vi "HMI_Prototype.vi"() -> ()   [LabVIEW 2015]
uses:
  System.Windows.Forms
  machineState.ctl
  controls.ctl
  <vilib>/DAQmx/write.llb/DAQmx Write (Digital Bool 1Line 1Point).vi
  <vilib>/DAQmx/read.llb/DAQmx Read (Analog DBL 1Chan 1Samp).vi
  <vilib>/DAQmx/miscellaneous.llb/DAQmx Fill In Error Info.vi
panel:
  out "lab":dbl
  out "solution":dbl
  out "Issue Resolved:":bool
  out "Budget:":dbl=800.0 format="$%#_g.00"
  out "Time Remaining:":timestamp=timestamp(1800 s since 1904-01-01) format="%<%M:%S>T"
  in  "Terminal:":T1(ring)
  in  "Component:":T2(ring)
  in  "Tighten Terminal":bool
  in  "Replace Component":bool
  in  "Segment:":T3(ring)
  in  "Aquire Voltage":bool
  out "Voltage:":dbl
  out "Lab:":string
  in  "Close Lab":bool
  in  "Reset Lab":bool
  out "B+ Solenoid":bool
  out "A- Solenoid":bool
  out "A+ Solenoid":bool
  out "Manual":bool
  out "Auto":bool=TRUE
  out "Stop Button":bool
  out "Start Button":bool
  in  "Tab Control":T4(tab)
  in  "WebBrowser":refnum<k7>(container)
  in  "Schematic1":refnum<k24>(container)
  in  "Schematic2":refnum<k24>(container)
  in  "Schematic3":refnum<k24>(container)
  in  "Schematic4":refnum<k24>(container)
  in  "B+":bool
  in  "A-":bool
  in  "A+":bool
  in  "START":bool
  in  "AUTO/MAN":bool
  in  "STOP":bool
  # "A+"
  # "A-"
  # "B+"
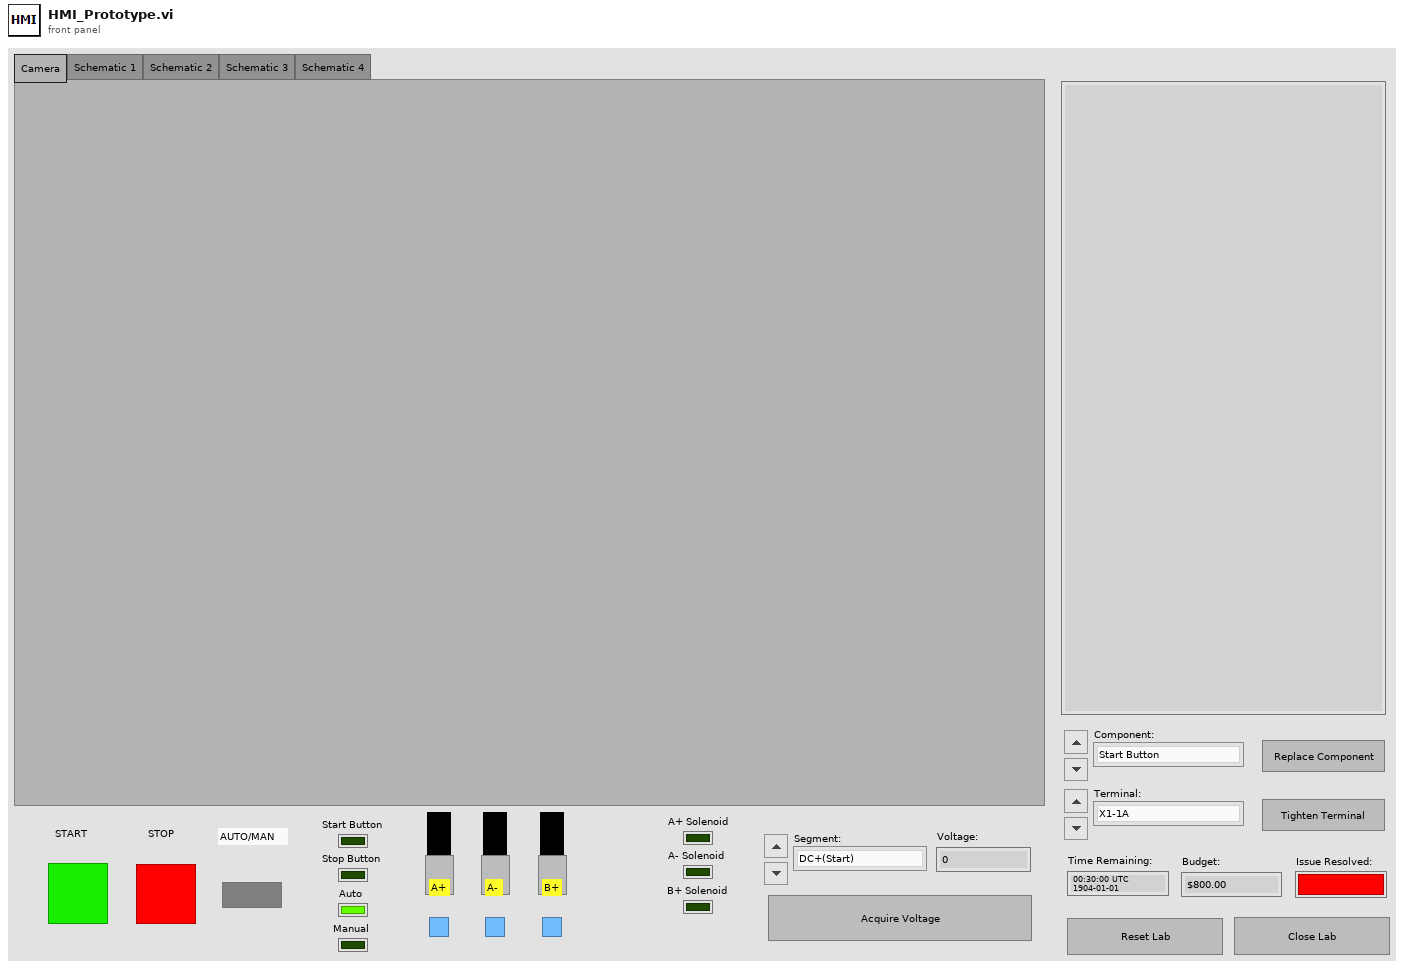
[diagram p1: front panel]
types:
  T1 = enum16{"X1-1A", "X1-2A", "X1-3A", "X1-4A", "X1-5A", "X1-6A", "X1-7A", "X1-8A", "X1-9A", "X1-10A", "X1-11A", "X1-12A", "X1-1B", "X1-2B", "X1-3B", "X1-4B", "X1-5B", "X1-6B", "X1-7B", "X1-8B", "X1-9B", "X1-10B", "X1-11B", "X1-12B", "X1-1C", "X1-2C", "X1-3C", "X1-4C", "X1-5C", "X1-6C", "X1-7C", "X1-8C", "X1-9C", "X1-10C", "X1-11C", "X1-12C", "X1-1D", "X1-2D", "X1-3D", "X1-4D", "X1-5D", "X1-6D", "X1-7D", "X1-8D", "X1-9D", "X1-10D", "X1-11D", "X1-12D", "PLC-VDC(O/0)", "PLC-O/0", "PLC-VDC(O/1)", "PLC-O/1", "PLC-VDC(O/2)", "PLC-O/2", "PLC-VDC(O/3)", "PLC-O/3", "PLC-DC_COM1", "PLC-I/0", "PLC-I/1", "PLC-I/2", "PLC-I/3", "PLC-DC_COM2", "PLC-I/4", "PLC-I/5", "PLC-I/6", "PLC-I/7", "Start Button Terminals", "Stop Button Terminals", "Auto/Man Terminals", "DM1(a0) Terminals", "DM2(a1) Terminals", "DM3(b0) Terminals", "DM4(b1) Terminals", "DM5(v) Terminals", "EL1(A+) Terminals", "EL2(A-) Terminals", "EL3(B+) Terminals", "EL4(V+) Terminals"}
  T2 = enum16{"Start Button", "Stop Button", "Auto/Man Switch", "DM1(a0)", "DM2(a1)", "DM3(b0)", "DM4(b1)", "DM5(v)", "EL1(A+)", "EL2(A-)", "EL3(B+)", "EL4(V+)", "PLC"}
  T3 = enum16{"DC+(Start)", "PB(Start)", "I/0(Start)", "DC+(Stop)", "PB(Stop)", "I/1(Stop)", "DC+(Auto/Man)", "I/2(Auto/Man)", "DC+(a0)", "I/3(a0)", "DC+(a1)", "I/4(a1)", "DC+(b0)", "I/5(b0)", "DC+(b1)", "I/6(b1)", "DC+(v)", "I/7(v)", "DC+(O/0)(VAC/VDC)", "O/0(EL1A+)", "EL1A+(A1)", "EL1A+(A2)", "DC+(O/1)(VAC/VDC)", "O/1(EL2A-)", "EL2A-(A1)", "EL2A-(A2)", "O/2(EL3B+)(A1)", "EL3B+(A2)", "O/3(EL4V+)(A1)", "EL4V+(A2)", "DC-(DC_COM)", "DC-(0V)"}
  T4 = enum32{"Camera", "Schematic 1", "Schematic 2", "Schematic 3", "Schematic 4"}
  T5 = typedef "controls.ctl" = enum16{"Initialize", "Start Button", "Stop Button", "AutoMan Switch", "A Plus Button", "A Minus Button", "B Plus Button", "V Plus Button", "Change View", "Acquire Voltage", "Replace Component", "Tighten Terminal", "Reset Lab", "Close Lab"}
  T6 = typedef "machineState.ctl" = enum16{"idle", "running"}
  T7 = enum16{"open", "replace", "create", "open or create", "replace or create", "replace or create with confirmation"}
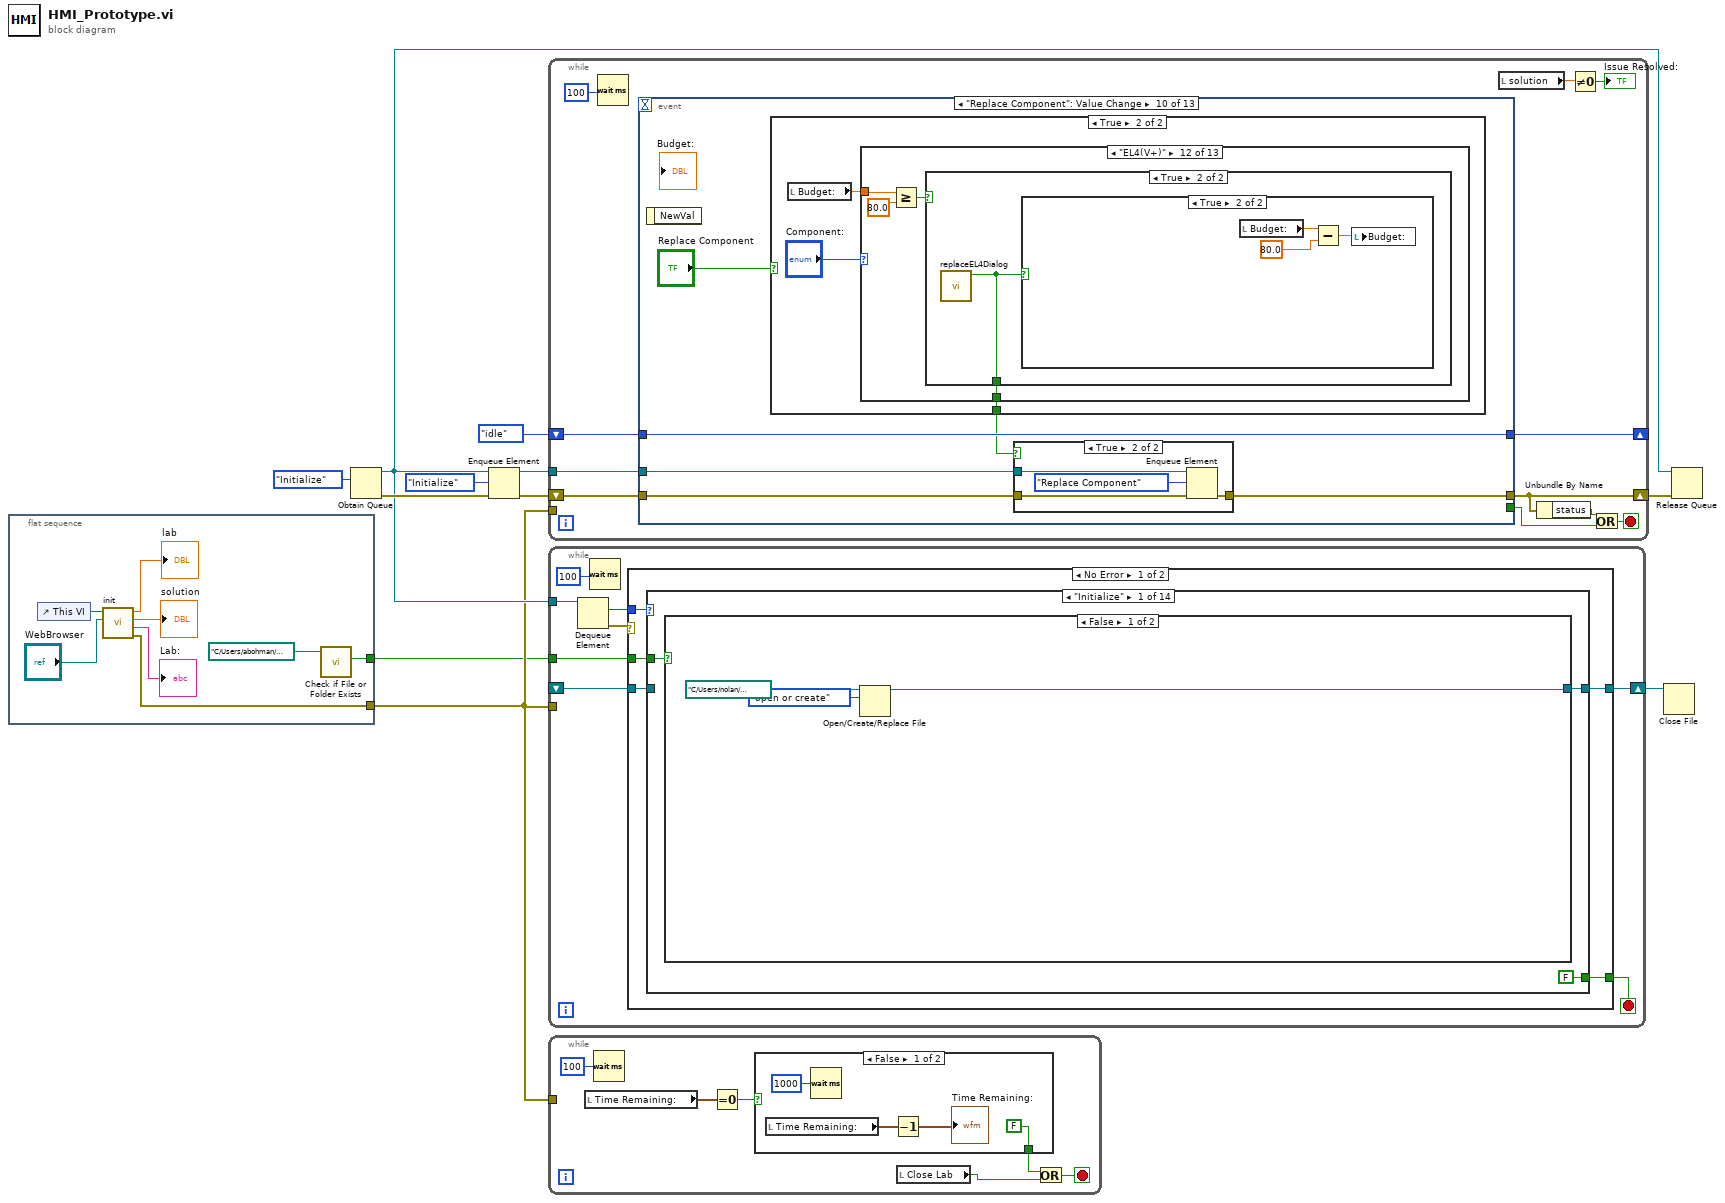
[diagram p0: block diagram]
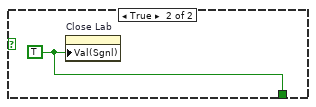
[diagram p2: hidden frame]
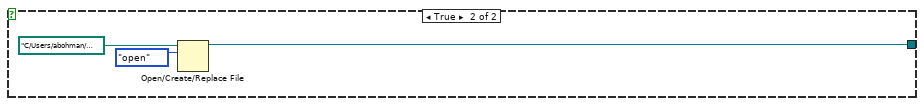
[diagram p3: hidden frame]
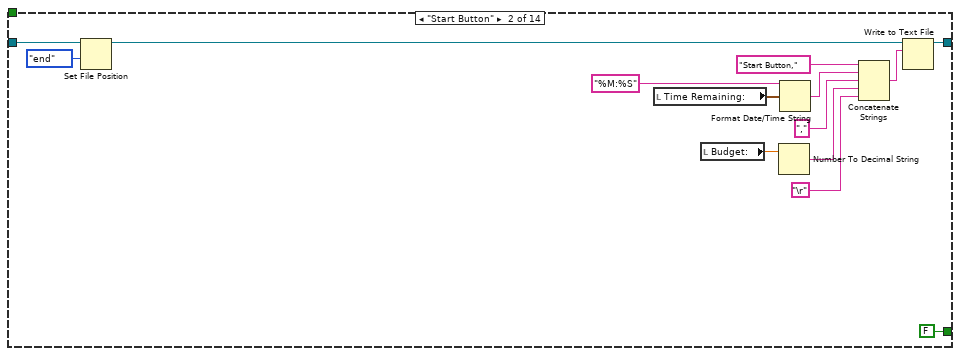
[diagram p4: hidden frame]
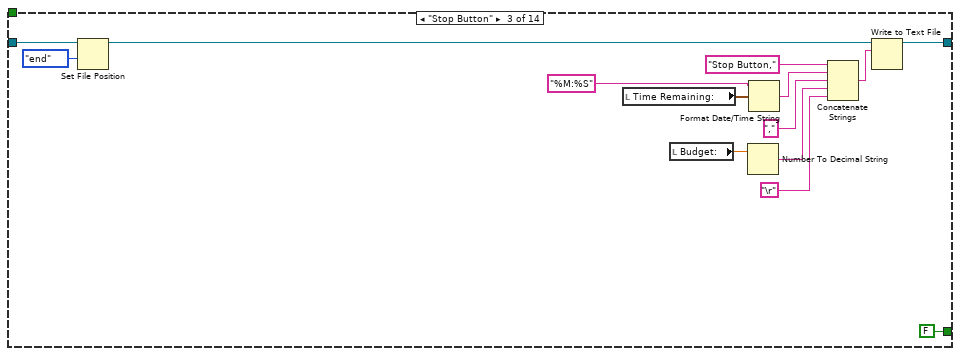
[diagram p5: hidden frame]
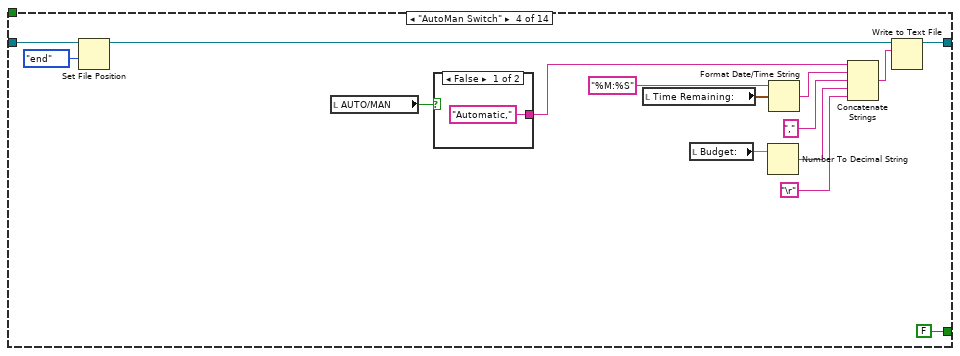
[diagram p6: hidden frame]
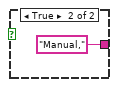
[diagram p7: hidden frame]
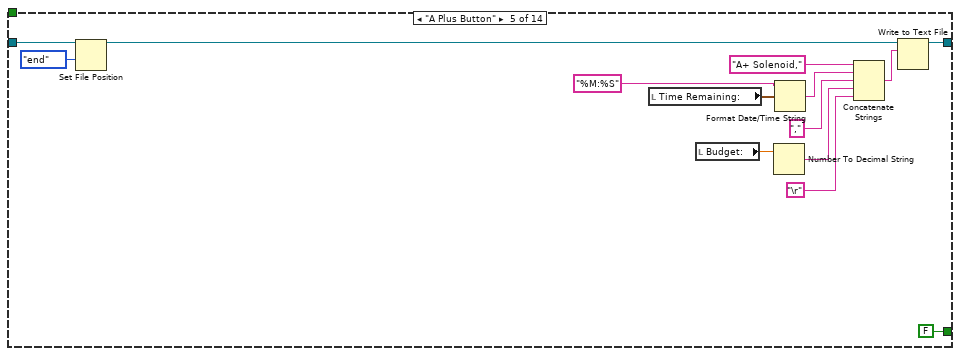
[diagram p8: hidden frame]
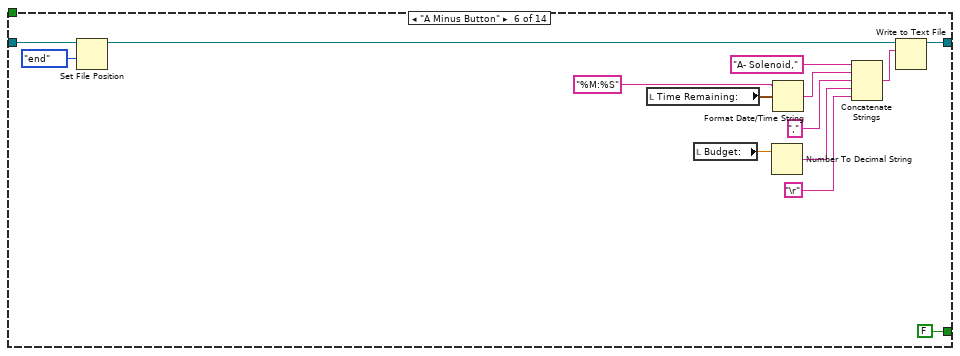
[diagram p9: hidden frame]
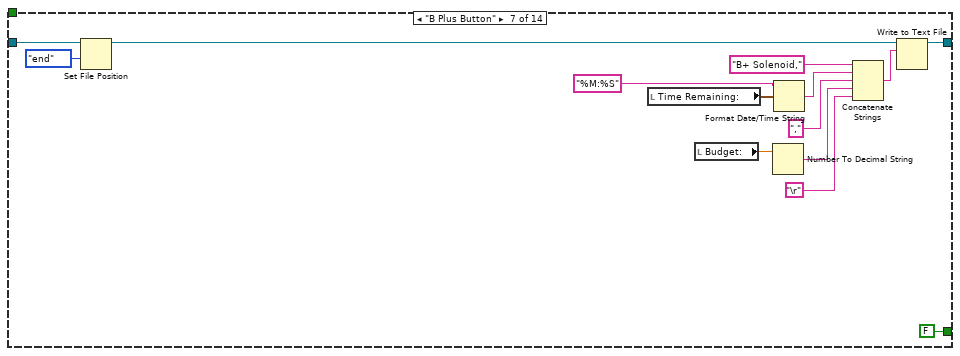
[diagram p10: hidden frame]
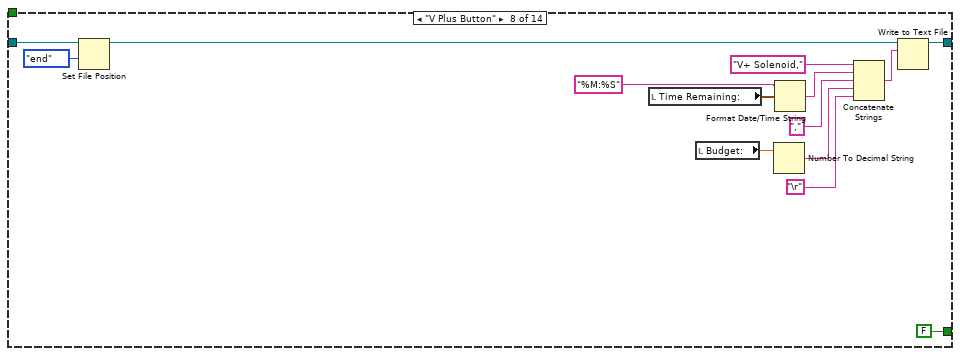
[diagram p11: hidden frame]
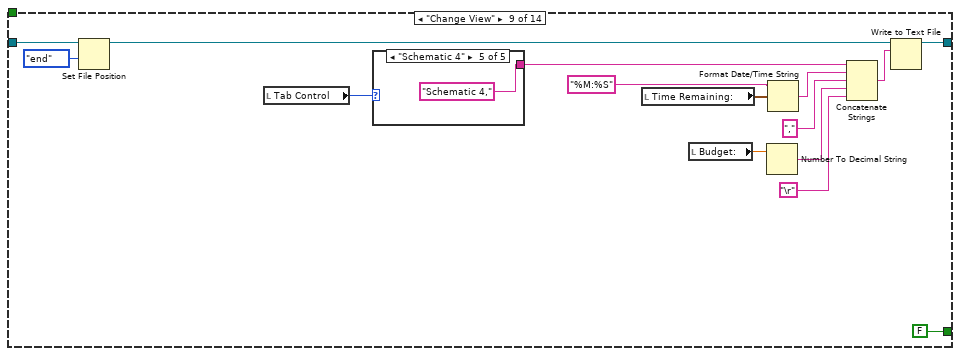
[diagram p12: hidden frame]
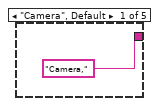
[diagram p13: hidden frame]
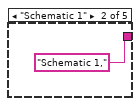
[diagram p14: hidden frame]
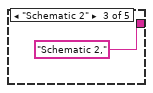
[diagram p15: hidden frame]
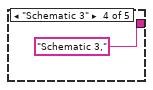
[diagram p16: hidden frame]
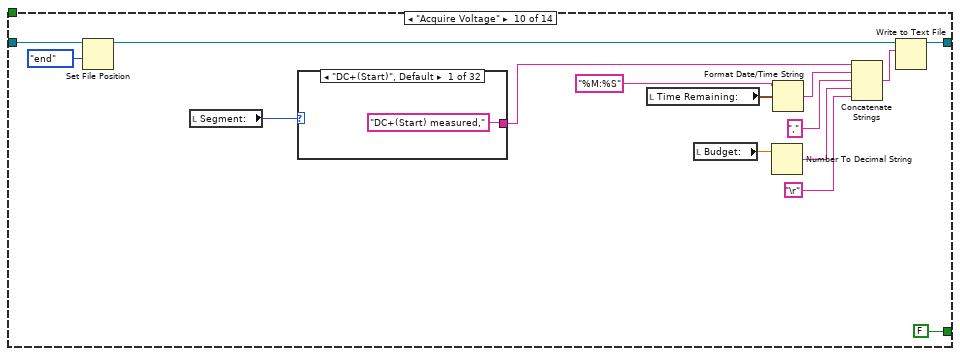
[diagram p17: hidden frame]
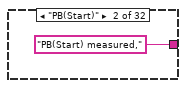
[diagram p18: hidden frame]
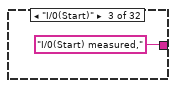
[diagram p19: hidden frame]
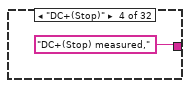
[diagram p20: hidden frame]
diagram:
  n1 = flat-sequence {
    tunnel: [w14] -> w3
    tunnel: [w12] -> w2
    frame #0 {
      n2 = control-ref of="This VI"() -> (w19:refnum<vi>)
      n3 = call "init.vi"("WebBrowser"="WebBrowser", "VI in"=w19) -> ("error out"=w14:errorcluster, "Lab Description:"=→"Lab:":string, "solution"=→"solution":dbl, "lab"=→"lab":dbl)  [unwired: 6 in]
      n4 = call <vilib>:"Check if File or Folder Exists.vi"("path"=path "C:/Users/abohman/Desktop/iMEC-HMI/userLog.txt") -> ("file or folder exists?"=w12:bool)  [unwired: 8 in, 2 out]
    }
  }
  n5 = Obtain Queue(element data type=controls."Initialize") -> (queue out=w4:refnum<queue>, error out=w5:errorcluster)  [unwired: 4 in, 1 out]
  n6 = Enqueue Element(queue=w4, element=controls."Initialize", error in (no error)=w5) -> (queue out=w8:refnum<queue>, error out=w7:errorcluster)  [unwired: 1 in, 1 out]
  n7 = while {
    shift-right: [w25] -> w10
    shift-left: w7 -> [w29]
    tunnel: w8 -> [w28]
    shift-right: [w26] -> _
    shift-left: machineState."idle" -> [w27]
    tunnel: w3 -> [_]
    stop <- w24 stop-if-true
    n8 = Wait (ms)(milliseconds to wait=u32 100 ("millisecond timer value")) -> ()  [unwired: 1 out]
    n9 = event shown="[9] \"Replace Component\": Value Change" {
      selector: _ -> [_ _ _ _ _ _ _ _ _ _ _ _ _]
      dyn-events: _ -> [_ _ _ _ _ _ _ _ _ _ _ _ _]
      timeout: _ -> [_ _ _ _ _ _ _ _ _ _ _ _ _]
      tunnel: w29 -> [w42 w69 w78 w91 w106 w122 w137 w142 w189 w195 w405 w516 w547]
      tunnel: [w41 w68 w79 w90 w105 w121 w136 w141 w189 w194 w404 w515 w545] -> w25
      tunnel: w28 -> [w40 w67 w77 w92 w107 w120 w138 w143 _ w196 w406 w517 w546]
      tunnel: w27 -> [w34 w64 w81 w89 w104 w119 w134 w140 w190 w193 w403 w514 w543]
      tunnel: [w35 w63 w81 w89 w104 w119 w134 w140 w190 w193 w403 w514 w543] -> w26
      tunnel: [_ _ _ _ _ _ _ _ _ _ _ _ w541] -> w22
      event "START": Value Change {
        w37 = refnum<k21> "DO1P0"  # Start Button
        n10 = event-data() -> ("NewVal"=w31:bool)  [unwired: 1 in]
        n11 = local read "AUTO/MAN"() -> (w39:bool)
        n12 = case shown="True" w31 {
          tunnel: w42 -> [w43 w47]
          tunnel: [w43 w46] -> w41
          tunnel: w40 -> [_ w45]
          frame False {
          }
          frame True {
            n13 = Enqueue Element(queue=w45, element=controls."Start Button", error in (no error)=w47) -> (error out=w46:errorcluster)  [unwired: 1 in, 2 out]
          }
        }
        n14 = case shown="False" w39 {
          tunnel: [w50 w60] -> w36
          tunnel: [w51 w59] -> w35
          tunnel: w34 -> [w52 w59]
          tunnel: "START" -> [w48 w60]
          tunnel: [w49 w60] -> w32
          frame False {
            n15 = case shown="\"idle\"" w52 {
              selector: w52 -> [_ w58]
              tunnel: [machineState."running" w58] -> w51
              tunnel: [TRUE ("START") FALSE ("START")] -> w50
              tunnel: [w53 w56] -> w49
              tunnel: w48 -> [w53 w56]
              frame "idle" {
              }
              frame "running" {
              }
            }
          }
          frame True {
          }
        }
        "Start Button" <- w32
        n16 = call-poly <vilib>:"DAQmx Write.vi"("task/channels in"=w37, "data"=w36) -> ("task out"=w38:refnum<k21>)  [unwired: 11 in, 2 out]
        n17 = call <vilib>:"DAQmx Clear Task.vi"("task in"=w38) -> ()  [unwired: 14 in, 1 out]
      }
      event "STOP": Value Change {
        w65 = refnum<k21> "DO1P1"  # Stop Button
        n18 = event-data() -> ("NewVal"=w62:bool)  [unwired: 1 in]
        n19 = case shown="True" w62 {
          tunnel: w69 -> [w70 w74]
          tunnel: [w70 w73] -> w68
          tunnel: w67 -> [_ w72]
          frame False {
          }
          frame True {
            n20 = Enqueue Element(queue=w72, element=controls."Stop Button", error in (no error)=w74) -> (error out=w73:errorcluster)  [unwired: 1 in, 2 out]
          }
        }
        n21 = case shown="\"running\"" w64 {
          selector: w64 -> [w75 _]
          tunnel: [w75 machineState."idle"] -> w63
          frame "idle" {
          }
          frame "running" {
          }
        }
        n22 = call-poly <vilib>:"DAQmx Write.vi"("task/channels in"=w65, "data"="STOP") -> ("task out"=w66:refnum<k21>)  [unwired: 11 in, 2 out]
        n23 = call <vilib>:"DAQmx Clear Task.vi"("task in"=w66) -> ()  [unwired: 14 in, 1 out]
        "Stop Button" <- "STOP"
      }
      event "AUTO/MAN": Value Change {
        n24 = event-data() -> ()  [unwired: 1 in, 1 out]
        n25 = case shown="\"idle\"" w81 {
          frame "idle" {
            w83 = refnum<k21> "DO1P2"  # Auto/Man
            n26 = Equal?(x="AUTO/MAN", y=FALSE) -> (x = y?=→"Auto":bool)
            n27 = call-poly <vilib>:"DAQmx Write.vi"("task/channels in"=w83, "data"="AUTO/MAN") -> ("task out"=w84:refnum<k21>)  [unwired: 11 in, 2 out]
            n28 = call <vilib>:"DAQmx Clear Task.vi"("task in"=w84) -> ()  [unwired: 14 in, 1 out]
            "Manual" <- "AUTO/MAN"
          }
          frame "running" {
            n29 = One Button Dialog(message="The machine is still running.  Please\nstop the machine before switching\nit into 'Manual' mode." ("button name (\"OK\")")) -> ()  [unwired: 1 in, 1 out]
            n30 = invoke on="AUTO/MAN" class="Bool (strict)" method="Reinit To Default"() -> ()  [unwired: 3 in, 3 out]
          }
        }
        n31 = Enqueue Element(queue=w77, element=controls."AutoMan Switch", error in (no error)=w78) -> (error out=w79:errorcluster)  [unwired: 1 in, 2 out]
      }
      event "A+": Value Change {
        n32 = event-data() -> ("NewVal"=w88:bool)  [unwired: 1 in]
        n33 = case shown="True" w88 {
          tunnel: w92 -> [_ w97]
          tunnel: w91 -> [w93 w96]
          tunnel: [w93 w95] -> w90
          frame False {
          }
          frame True {
            n34 = Enqueue Element(queue=w97, element=controls."A Plus Button", error in (no error)=w96) -> (error out=w95:errorcluster)  [unwired: 1 in, 2 out]
          }
        }
        n35 = case shown="\"idle\"" w89 {
          frame "idle" {
            w99 = refnum<k21> "DO1P3"  # A+ Solenoid
            n36 = call-poly <vilib>:"DAQmx Write.vi"("task/channels in"=w99, "data"="A+") -> ("task out"=w100:refnum<k21>)  [unwired: 11 in, 2 out]
            n37 = call <vilib>:"DAQmx Clear Task.vi"("task in"=w100) -> ()  [unwired: 14 in, 1 out]
            "A+ Solenoid" <- "A+"
          }
          frame "running" {
            n38 = local read "A+"() -> (w101:bool)
            n39 = case shown="True" w101 {
              frame False {
              }
              frame True {
                n40 = One Button Dialog(message="The machine is still running. Please\nstop the machine before using\nthe solenoid controls.") -> ()  [unwired: 1 in, 1 out]
              }
            }
          }
        }
      }
      event "A-": Value Change {
        n41 = event-data() -> ("NewVal"=w103:bool)  [unwired: 1 in]
        n42 = case shown="True" w103 {
          tunnel: w107 -> [_ w112]
          tunnel: w106 -> [w108 w111]
          tunnel: [w108 w110] -> w105
          frame False {
          }
          frame True {
            n43 = Enqueue Element(queue=w112, element=controls."A Minus Button", error in (no error)=w111) -> (error out=w110:errorcluster)  [unwired: 1 in, 2 out]
          }
        }
        n44 = case shown="\"idle\"" w104 {
          frame "idle" {
            w114 = refnum<k21> "DO1P4"  # A- Solenoid
            n45 = call-poly <vilib>:"DAQmx Write.vi"("task/channels in"=w114, "data"="A-") -> ("task out"=w115:refnum<k21>)  [unwired: 11 in, 2 out]
            n46 = call <vilib>:"DAQmx Clear Task.vi"("task in"=w115) -> ()  [unwired: 14 in, 1 out]
            "A- Solenoid" <- "A-"
          }
          frame "running" {
            n47 = local read "A-"() -> (w116:bool)
            n48 = case shown="True" w116 {
              frame False {
              }
              frame True {
                n49 = One Button Dialog(message="The machine is still running. Please\nstop the machine before using\nthe solenoid controls.") -> ()  [unwired: 1 in, 1 out]
              }
            }
          }
        }
      }
      event "B+": Value Change {
        n50 = event-data() -> ("NewVal"=w118:bool)  [unwired: 1 in]
        n51 = case shown="True" w118 {
          tunnel: w122 -> [w123 w127]
          tunnel: [w123 w126] -> w121
          tunnel: w120 -> [_ w125]
          frame False {
          }
          frame True {
            n52 = Enqueue Element(queue=w125, element=controls."B Plus Button", error in (no error)=w127) -> (error out=w126:errorcluster)  [unwired: 1 in, 2 out]
          }
        }
        n53 = case shown="\"running\"" w119 {
          frame "idle" {
            w129 = refnum<k21> "DO1P5"  # B+ Solenoid
            n54 = call-poly <vilib>:"DAQmx Write.vi"("task/channels in"=w129, "data"="B+") -> ("task out"=w130:refnum<k21>)  [unwired: 11 in, 2 out]
            n55 = call <vilib>:"DAQmx Clear Task.vi"("task in"=w130) -> ()  [unwired: 14 in, 1 out]
            "B+ Solenoid" <- "B+"
          }
          frame "running" {
            n56 = local read "B+"() -> (w131:bool)
            n57 = case shown="True" w131 {
              frame False {
              }
              frame True {
                n58 = One Button Dialog(message="The machine is still running. Please\nstop the machine before using\nthe solenoid controls.") -> ()  [unwired: 1 in, 1 out]
              }
            }
          }
        }
      }
      event "Tab Control": Value Change {
        n59 = event-data() -> ()  [unwired: 1 in, 1 out]
        n60 = case shown="\"Schematic 1\"" "Tab Control" {
          frame "Camera", Default {
          }
          frame "Schematic 1" {
          }
          frame "Schematic 2" {
          }
          frame "Schematic 3" {
          }
          frame "Schematic 4" {
          }
        }
        n61 = Enqueue Element(queue=w138, element=controls."Change View", error in (no error)=w137) -> (error out=w136:errorcluster)  [unwired: 1 in, 2 out]
      }
      event "Aquire Voltage": Value Change {
        n62 = event-data() -> ("NewVal"=w139:bool)  [unwired: 1 in]
        n63 = while {
          stop <- w149 stop-if-true
          n64 = case shown="True" "Aquire Voltage" {
            tunnel: [TRUE FALSE] -> w149
            frame False {
            }
            frame True {
              n65 = case shown="\"DC-(DC_COM)\"" "Segment:" {
                tunnel: [w157 w158 w159 w160 w161 w162 w163 w164 w165 w166 w167 w168 w169 w170 w171 w172 w173 w174 w175 w176 w177 w178 w179 w180 w181 w182 w183 w184 w185 w186 w187 w188] -> w154
                frame "DC+(Start)" {
                  w157 = refnum<k21> "ACH00"  # DC+(Start)
                }
                frame "PB(Start)" {
                  w158 = refnum<k21> "ACH01"  # PB(Start)
                }
                frame "I/0(Start)" {
                  w159 = refnum<k21> "ACH02"  # I/0(Start)
                }
                frame "DC+(Stop)" {
                  w160 = refnum<k21> "ACH03"  # DC+(Stop)
                }
                frame "PB(Stop)" {
                  w161 = refnum<k21> "ACH04"  # PB(Stop)
                }
                frame "I/1(Stop)" {
                  w162 = refnum<k21> "ACH05"  # I/1(Stop)
                }
                frame "DC+(Auto/Man)" {
                  w163 = refnum<k21> "ACH06"  # DC+(Auto/Man)
                }
                frame "I/2(Auto/Man)" {
                  w164 = refnum<k21> "ACH07"  # I/2(Auto/Man)
                }
                frame "DC+(a0)" {
                  w165 = refnum<k21> "ACH08"  # DC+(A0)
                }
                frame "I/3(a0)" {
                  w166 = refnum<k21> "ACH09"  # I/3(A0)
                }
                frame "DC+(a1)" {
                  w167 = refnum<k21> "ACH10"  # DC+(A1)
                }
                frame "I/4(a1)" {
                  w168 = refnum<k21> "ACH11"  # I/4(A1)
                }
                frame "DC+(b0)" {
                  w169 = refnum<k21> "ACH12"  # DC+(B0)
                }
                frame "I/5(b0)" {
                  w170 = refnum<k21> "ACH13"  # I/5(B0)
                }
                frame "DC+(b1)" {
                  w171 = refnum<k21> "ACH14"  # DC+(B1)
                }
                frame "I/6(b1)" {
                  w172 = refnum<k21> "ACH15"  # I/6(B1)
                }
                frame "DC+(v)" {
                  w173 = refnum<k21> "ACH16"  # DC+(V)
                }
                frame "I/7(v)" {
                  w174 = refnum<k21> "ACH17"  # I/7(V)
                }
                frame "DC+(O/0)(VAC/VDC)" {
                  w175 = refnum<k21> "ACH18"  # DC+(O/0)(VAC/VDC)
                }
                frame "O/0(EL1A+)" {
                  w176 = refnum<k21> "ACH19"  # O/0(EL1A+)
                }
                frame "EL1A+(A1)" {
                  w177 = refnum<k21> "ACH20"  # EL1A+(A1)
                }
                frame "EL1A+(A2)" {
                  w178 = refnum<k21> "ACH21"  # EL1A+(A2)
                }
                frame "DC+(O/1)(VAC/VDC)" {
                  w179 = refnum<k21> "ACH22"  # DC+(O/1)(VAC/VDC)
                }
                frame "O/1(EL2A-)" {
                  w180 = refnum<k21> "ACH23"  # O/1(EL2A-)
                }
                frame "EL2A-(A1)" {
                  w181 = refnum<k21> "ACH24"  # EL2A-(A1)
                }
                frame "EL2A-(A2)" {
                  w182 = refnum<k21> "ACH25"  # EL2A-(A2)
                }
                frame "O/2(EL3B+)(A1)" {
                  w183 = refnum<k21> "ACH26"  # O/2(EL3B+)(A1)
                }
                frame "EL3B+(A2)" {
                  w184 = refnum<k21> "ACH27"  # EL3B+(A2)
                }
                frame "O/3(EL4V+)(A1)" {
                  w185 = refnum<k21> "ACH28"  # O/3(EL4V+)(A1)
                }
                frame "EL4V+(A2)" {
                  w186 = refnum<k21> "ACH29"  # EL4V+(A2)
                }
                frame "DC-(DC_COM)" {
                  w187 = refnum<k21> "ACH30"  # DC-(DC_COM)
                }
                frame "DC-(0V)" {
                  w188 = refnum<k21> "ACH31"  # DC-(0V)
                }
              }
              n66 = call-poly <vilib>:"DAQmx Read.vi"("task/channels in"=w154) -> ("task out"=w155:refnum<k21>, "data"=→"Voltage:":dbl)  [unwired: 12 in, 1 out]
              n67 = call <vilib>:"DAQmx Clear Task.vi"("task in"=w155) -> ()  [unwired: 14 in, 1 out]
            }
          }
        }
        n68 = case shown="True" w139 {
          tunnel: w143 -> [_ w148]
          tunnel: w142 -> [w144 w147]
          tunnel: [w144 w146] -> w141
          frame False {
          }
          frame True {
            n69 = Enqueue Element(queue=w148, element=controls."Acquire Voltage", error in (no error)=w147) -> (error out=w146:errorcluster)  [unwired: 1 in, 2 out]
          }
        }
      }
      event "Segment:": Value Change {
        n70 = event-data() -> ()  [unwired: 1 in, 1 out]
        n71 = invoke on="Voltage:" class="DigNum (strict)" method="Reinit To Default"() -> ()  [unwired: 3 in, 3 out]
      }
      event "Replace Component": Value Change {
        n72 = event-data() -> ()  [unwired: 1 in, 1 out]
        n73 = case shown="True" "Replace Component" {
          tunnel: [FALSE ("T button?") w203] -> w191
          frame False {
          }
          frame True {
            n74 = local read "Budget:"() -> (w204:dbl)
            n75 = case shown="\"EL4(V+)\"" "Component:" {
              tunnel: w204 -> [w209 w228 w247 w257 w266 w285 w304 w314 w324 w343 w353 w372 w382]
              tunnel: [w206 w225 w244 w254 w264 w283 w302 w312 w322 w341 w351 w370 w380] -> w203
              frame "Start Button" {
                n76 = Greater Or Equal?(x=w209, y=20.0) -> (x >= y?=w207:bool)
                n77 = case shown="True" w207 {
                  tunnel: [FALSE ("T button?") w212] -> w206
                  frame False {
                    n78 = One Button Dialog(message="You don't have enough money left in the budget.") -> ()  [unwired: 1 in, 1 out]
                  }
                  frame True {
                    n79 = call "replaceStartDialog.vi"() -> ("T button?"=w212:bool)  [unwired: 11 in]
                    n80 = case shown="True" w212 {
                      frame False {
                      }
                      frame True {
                        n81 = local read "Budget:"() -> (w223:dbl)
                        n82 = local read "solution"() -> (w221:dbl)
                        n83 = local read "lab"() -> (w214:dbl)
                        n84 = Subtract(x=w223, y=20.0) -> (x-y=w224:dbl)
                        n85 = Equal To 0?(x=w221) -> (x = 0?=w216:bool)
                        n86 = Equal?(x=w214, y=1.0) -> (x = y?=w215:bool)
                        n87 = local write "Budget:"(w224) -> ()
                        n88 = And(x=w216, y=w215) -> (x .and. y?=w217:bool)
                        n89 = local read "solution"() -> (w218:dbl)
                        n90 = call "turnOffFault1.vi"() -> ()  [unwired: 12 in]
                        n91 = Select(t=1.0, s=w217, f=w218) -> (s? t:f=w219:dbl)
                        n92 = local write "solution"(w219) -> ()
                      }
                    }
                  }
                }
              }
              frame "Stop Button" {
                n93 = Greater Or Equal?(x=w228, y=20.0) -> (x >= y?=w226:bool)
                n94 = case shown="True" w226 {
                  tunnel: [FALSE ("T button?") w231] -> w225
                  frame False {
                    n95 = One Button Dialog(message="You don't have enough money left in the budget.") -> ()  [unwired: 1 in, 1 out]
                  }
                  frame True {
                    n96 = call "replaceStopDialog.vi"() -> ("T button?"=w231:bool)  [unwired: 11 in]
                    n97 = case shown="True" w231 {
                      frame False {
                      }
                      frame True {
                        n98 = local read "Budget:"() -> (w243:dbl)
                        n99 = local read "solution"() -> (w240:dbl)
                        n100 = local read "lab"() -> (w233:dbl)
                        n101 = Subtract(x=w243, y=20.0) -> (x-y=w241:dbl)
                        n102 = Equal To 0?(x=w240) -> (x = 0?=w235:bool)
                        n103 = Equal?(x=w233, y=3.0) -> (x = y?=w234:bool)
                        n104 = local write "Budget:"(w241) -> ()
                        n105 = And(x=w235, y=w234) -> (x .and. y?=w236:bool)
                        n106 = local read "solution"() -> (w237:dbl)
                        n107 = Select(t=1.0, s=w236, f=w237) -> (s? t:f=w238:dbl)
                        n108 = call "turnOffFault3.vi"() -> ()  [unwired: 12 in]
                        n109 = local write "solution"(w238) -> ()
                      }
                    }
                  }
                }
              }
              frame "Auto/Man Switch" {
                n110 = Greater Or Equal?(x=w247, y=30.0) -> (x >= y?=w245:bool)
                n111 = case shown="True" w245 {
                  tunnel: [FALSE ("T button?") w250] -> w244
                  frame False {
                    n112 = One Button Dialog(message="You don't have enough money left in the budget.") -> ()  [unwired: 1 in, 1 out]
                  }
                  frame True {
                    n113 = call "replaceAutoManDialog.vi"() -> ("T button?"=w250:bool)  [unwired: 11 in]
                    n114 = case shown="True" w250 {
                      frame False {
                      }
                      frame True {
                        n115 = local read "Budget:"() -> (w252:dbl)
                        n116 = Subtract(x=w252, y=30.0) -> (x-y=w251:dbl)
                        n117 = local write "Budget:"(w251) -> ()
                      }
                    }
                  }
                }
              }
              frame "DM1(a0)" {
                n118 = Greater Or Equal?(x=w257, y=120.0) -> (x >= y?=w255:bool)
                n119 = case shown="True" w255 {
                  tunnel: [FALSE ("T button?") w260] -> w254
                  frame False {
                    n120 = One Button Dialog(message="You don't have enough money left in the budget.") -> ()  [unwired: 1 in, 1 out]
                  }
                  frame True {
                    n121 = call "replaceDM1Dialog.vi"() -> ("T button?"=w260:bool)  [unwired: 11 in]
                    n122 = case shown="True" w260 {
                      frame False {
                      }
                      frame True {
                        n123 = local read "Budget:"() -> (w262:dbl)
                        n124 = Subtract(x=w262, y=120.0) -> (x-y=w261:dbl)
                        n125 = local write "Budget:"(w261) -> ()
                      }
                    }
                  }
                }
              }
              frame "DM2(a1)" {
                n126 = Greater Or Equal?(x=w266, y=120.0) -> (x >= y?=w265:bool)
                n127 = case shown="True" w265 {
                  tunnel: [FALSE ("T button?") w270] -> w264
                  frame False {
                    n128 = One Button Dialog(message="You don't have enough money left in the budget.") -> ()  [unwired: 1 in, 1 out]
                  }
                  frame True {
                    n129 = call "replaceDM2Dialog.vi"() -> ("T button?"=w270:bool)  [unwired: 11 in]
                    n130 = case shown="True" w270 {
                      frame False {
                      }
                      frame True {
                        n131 = local read "solution"() -> (w271:dbl)
                        n132 = local read "lab"() -> (w278:dbl)
                        n133 = local read "Budget:"() -> (w281:dbl)
                        n134 = Equal To 0?(x=w271) -> (x = 0?=w276:bool)
                        n135 = Equal?(x=w278, y=4.0) -> (x = y?=w277:bool)
                        n136 = Subtract(x=w281, y=120.0) -> (x-y=w280:dbl)
                        n137 = And(x=w276, y=w277) -> (x .and. y?=w275:bool)
                        n138 = local read "solution"() -> (w274:dbl)
                        n139 = local write "Budget:"(w280) -> ()
                        n140 = Select(t=1.0, s=w275, f=w274) -> (s? t:f=w273:dbl)
                        n141 = call "turnOffFault4.vi"() -> ()  [unwired: 12 in]
                        n142 = local write "solution"(w273) -> ()
                      }
                    }
                  }
                }
              }
              frame "DM3(b0)" {
                n143 = Greater Or Equal?(x=w285, y=120.0) -> (x >= y?=w284:bool)
                n144 = case shown="True" w284 {
                  tunnel: [FALSE ("T button?") w289] -> w283
                  frame False {
                    n145 = One Button Dialog(message="You don't have enough money left in the budget.") -> ()  [unwired: 1 in, 1 out]
                  }
                  frame True {
                    n146 = call "replaceDM3Dialog.vi"() -> ("T button?"=w289:bool)  [unwired: 11 in]
                    n147 = case shown="True" w289 {
                      frame False {
                      }
                      frame True {
                        n148 = local read "solution"() -> (w290:dbl)
                        n149 = local read "lab"() -> (w297:dbl)
                        n150 = local read "Budget:"() -> (w300:dbl)
                        n151 = Equal To 0?(x=w290) -> (x = 0?=w295:bool)
                        n152 = Equal?(x=w297, y=2.0) -> (x = y?=w296:bool)
                        n153 = Subtract(x=w300, y=120.0) -> (x-y=w299:dbl)
                        n154 = And(x=w295, y=w296) -> (x .and. y?=w294:bool)
                        n155 = local read "solution"() -> (w293:dbl)
                        n156 = local write "Budget:"(w299) -> ()
                        n157 = Select(t=3.0, s=w294, f=w293) -> (s? t:f=w292:dbl)
                        n158 = call "turnOffFault2.vi"() -> ()  [unwired: 12 in]
                        n159 = local write "solution"(w292) -> ()
                      }
                    }
                  }
                }
              }
              frame "DM4(b1)" {
                n160 = Greater Or Equal?(x=w304, y=120.0) -> (x >= y?=w303:bool)
                n161 = case shown="True" w303 {
                  tunnel: [FALSE ("T button?") w308] -> w302
                  frame False {
                    n162 = One Button Dialog(message="You don't have enough money left in the budget.") -> ()  [unwired: 1 in, 1 out]
                  }
                  frame True {
                    n163 = call "replaceDM4Dialog.vi"() -> ("T button?"=w308:bool)  [unwired: 11 in]
                    n164 = case shown="True" w308 {
                      frame False {
                      }
                      frame True {
                        n165 = local read "Budget:"() -> (w310:dbl)
                        n166 = Subtract(x=w310, y=120.0) -> (x-y=w309:dbl)
                        n167 = local write "Budget:"(w309) -> ()
                      }
                    }
                  }
                }
              }
              frame "DM5(v)" {
                n168 = Greater Or Equal?(x=w314, y=120.0) -> (x >= y?=w313:bool)
                n169 = case shown="True" w313 {
                  tunnel: [FALSE ("T button?") w318] -> w312
                  frame False {
                    n170 = One Button Dialog(message="You don't have enough money left in the budget.") -> ()  [unwired: 1 in, 1 out]
                  }
                  frame True {
                    n171 = call "replaceDM5Dialog.vi"() -> ("T button?"=w318:bool)  [unwired: 11 in]
                    n172 = case shown="True" w318 {
                      frame False {
                      }
                      frame True {
                        n173 = local read "Budget:"() -> (w319:dbl)
                        n174 = Subtract(x=w319, y=120.0) -> (x-y=w321:dbl)
                        n175 = local write "Budget:"(w321) -> ()
                      }
                    }
                  }
                }
              }
              frame "EL1(A+)" {
                n176 = Greater Or Equal?(x=w324, y=80.0) -> (x >= y?=w323:bool)
                n177 = case shown="True" w323 {
                  tunnel: [FALSE ("T button?") w328] -> w322
                  frame False {
                    n178 = One Button Dialog(message="You don't have enough money left in the budget.") -> ()  [unwired: 1 in, 1 out]
                  }
                  frame True {
                    n179 = call "replaceEL1Dialog.vi"() -> ("T button?"=w328:bool)  [unwired: 11 in]
                    n180 = case shown="True" w328 {
                      frame False {
                      }
                      frame True {
                        n181 = local read "solution"() -> (w329:dbl)
                        n182 = local read "lab"() -> (w336:dbl)
                        n183 = local read "Budget:"() -> (w338:dbl)
                        n184 = Equal To 0?(x=w329) -> (x = 0?=w334:bool)
                        n185 = Equal?(x=w336, y=7.0) -> (x = y?=w335:bool)
                        n186 = Subtract(x=w338, y=80.0) -> (x-y=w340:dbl)
                        n187 = And(x=w334, y=w335) -> (x .and. y?=w333:bool)
                        n188 = local read "solution"() -> (w332:dbl)
                        n189 = local write "Budget:"(w340) -> ()
                        n190 = Select(t=1.0, s=w333, f=w332) -> (s? t:f=w331:dbl)
                        n191 = call "turnOffFault7.vi"() -> ()  [unwired: 12 in]
                        n192 = local write "solution"(w331) -> ()
                      }
                    }
                  }
                }
              }
              frame "EL2(A-)" {
                n193 = Greater Or Equal?(x=w343, y=80.0) -> (x >= y?=w342:bool)
                n194 = case shown="True" w342 {
                  tunnel: [FALSE ("T button?") w347] -> w341
                  frame False {
                    n195 = One Button Dialog(message="You don't have enough money left in the budget.") -> ()  [unwired: 1 in, 1 out]
                  }
                  frame True {
                    n196 = call "replaceEL2Dialog.vi"() -> ("T button?"=w347:bool)  [unwired: 11 in]
                    n197 = case shown="True" w347 {
                      frame False {
                      }
                      frame True {
                        n198 = local read "Budget:"() -> (w348:dbl)
                        n199 = Subtract(x=w348, y=80.0) -> (x-y=w350:dbl)
                        n200 = local write "Budget:"(w350) -> ()
                      }
                    }
                  }
                }
              }
              frame "EL3(B+)" {
                n201 = Greater Or Equal?(x=w353, y=80.0) -> (x >= y?=w352:bool)
                n202 = case shown="True" w352 {
                  tunnel: [FALSE ("T button?") w357] -> w351
                  frame False {
                    n203 = One Button Dialog(message="You don't have enough money left in the budget.") -> ()  [unwired: 1 in, 1 out]
                  }
                  frame True {
                    n204 = call "replaceEL3Dialog.vi"() -> ("T button?"=w357:bool)  [unwired: 11 in]
                    n205 = case shown="True" w357 {
                      frame False {
                      }
                      frame True {
                        n206 = local read "solution"() -> (w358:dbl)
                        n207 = local read "lab"() -> (w365:dbl)
                        n208 = local read "Budget:"() -> (w367:dbl)
                        n209 = Equal To 0?(x=w358) -> (x = 0?=w363:bool)
                        n210 = Equal?(x=w365, y=5.0) -> (x = y?=w364:bool)
                        n211 = Subtract(x=w367, y=80.0) -> (x-y=w369:dbl)
                        n212 = And(x=w363, y=w364) -> (x .and. y?=w362:bool)
                        n213 = local read "solution"() -> (w361:dbl)
                        n214 = local write "Budget:"(w369) -> ()
                        n215 = Select(t=3.0, s=w362, f=w361) -> (s? t:f=w360:dbl)
                        n216 = call "turnOffFault5.vi"() -> ()  [unwired: 12 in]
                        n217 = local write "solution"(w360) -> ()
                      }
                    }
                  }
                }
              }
              frame "EL4(V+)" {
                n218 = Greater Or Equal?(x=w372, y=80.0) -> (x >= y?=w371:bool)
                n219 = case shown="True" w371 {
                  tunnel: [FALSE ("T button?") w376] -> w370
                  frame False {
                    n220 = One Button Dialog(message="You don't have enough money left in the budget.") -> ()  [unwired: 1 in, 1 out]
                  }
                  frame True {
                    n221 = call "replaceEL4Dialog.vi"() -> ("T button?"=w376:bool)  [unwired: 11 in]
                    n222 = case shown="True" w376 {
                      frame False {
                      }
                      frame True {
                        n223 = local read "Budget:"() -> (w377:dbl)
                        n224 = Subtract(x=w377, y=80.0) -> (x-y=w379:dbl)
                        n225 = local write "Budget:"(w379) -> ()
                      }
                    }
                  }
                }
              }
              frame "PLC" {
                n226 = Greater Or Equal?(x=w382, y=600.0) -> (x >= y?=w381:bool)
                n227 = case shown="True" w381 {
                  tunnel: [FALSE ("T button?") w386] -> w380
                  frame False {
                    n228 = One Button Dialog(message="You don't have enough money left in the budget.") -> ()  [unwired: 1 in, 1 out]
                  }
                  frame True {
                    n229 = call "replacePLCDialog.vi"() -> ("T button?"=w386:bool)  [unwired: 11 in]
                    n230 = case shown="True" w386 {
                      frame False {
                      }
                      frame True {
                        n231 = local read "Budget:"() -> (w398:dbl)
                        n232 = local read "solution"() -> (w394:dbl)
                        n233 = local read "lab"() -> (w387:dbl)
                        n234 = Subtract(x=w398, y=600.0) -> (x-y=w400:dbl)
                        n235 = Or(x=6.0 ("y"), y=8.0) -> (x .or. y?=w395:i32)
                        n236 = Equal To 0?(x=w394) -> (x = 0?=w389:bool)
                        n237 = Equal?(x=w387, y=w395) -> (x = y?=w388:bool)
                        n238 = local write "Budget:"(w400) -> ()
                        n239 = And(x=w389, y=w388) -> (x .and. y?=w390:bool)
                        n240 = local read "solution"() -> (w391:dbl)
                        n241 = call "turnOffFault6.vi"() -> ()  [unwired: 12 in]
                        n242 = Select(t=1.0, s=w390, f=w391) -> (s? t:f=w392:dbl)
                        n243 = call "turnOffFault8.vi"() -> ()  [unwired: 12 in]
                        n244 = local write "solution"(w392) -> ()
                      }
                    }
                  }
                }
              }
            }
          }
        }
        n245 = case shown="True" w191 {
          tunnel: w196 -> [_ w201]
          tunnel: w195 -> [w197 w200]
          tunnel: [w197 w199] -> w194
          frame False {
          }
          frame True {
            n246 = Enqueue Element(queue=w201, element=controls."Replace Component", error in (no error)=w200) -> (error out=w199:errorcluster)  [unwired: 1 in, 2 out]
          }
        }
      }
      event "Tighten Terminal": Value Change {
        n247 = event-data() -> ("NewVal"=w401:bool)  [unwired: 1 in]
        n248 = case shown="True" w401 {
          tunnel: w406 -> [_ w411]
          tunnel: w405 -> [w407 w410]
          tunnel: [w407 w409] -> w404
          frame False {
          }
          frame True {
            n249 = Enqueue Element(queue=w411, element=controls."Tighten Terminal", error in (no error)=w410) -> (error out=w409:errorcluster)  [unwired: 1 in, 2 out]
          }
        }
        n250 = case shown="True" "Tighten Terminal" {
          frame False {
          }
          frame True {
            n251 = case shown="\"PLC-VDC(O/1)\"" "Terminal:" {
              frame "X1-1A" {
              }
              frame "X1-2A" {
              }
              frame "X1-3A" {
              }
              frame "X1-4A" {
              }
              frame "X1-5A" {
              }
              frame "X1-6A" {
              }
              frame "X1-7A" {
              }
              frame "X1-8A" {
              }
              frame "X1-9A" {
                n252 = call "turnOffFault7.vi"() -> ()  [unwired: 12 in]
                n253 = local read "solution"() -> (w413:dbl)
                n254 = local read "lab"() -> (w420:dbl)
                n255 = Equal To 0?(x=w413) -> (x = 0?=w418:bool)
                n256 = Equal?(x=w420, y=7.0) -> (x = y?=w419:bool)
                n257 = And(x=w418, y=w419) -> (x .and. y?=w417:bool)
                n258 = local read "solution"() -> (w416:dbl)
                n259 = Select(t=2.0, s=w417, f=w416) -> (s? t:f=w415:dbl)
                n260 = local write "solution"(w415) -> ()
              }
              frame "X1-10A" {
              }
              frame "X1-11A" {
              }
              frame "X1-12A" {
              }
              frame "X1-1B" {
                n261 = call "turnOffFault1.vi"() -> ()  [unwired: 12 in]
                n262 = local read "solution"() -> (w422:dbl)
                n263 = local read "lab"() -> (w429:dbl)
                n264 = Equal To 0?(x=w422) -> (x = 0?=w427:bool)
                n265 = Equal?(x=w429, y=1.0) -> (x = y?=w428:bool)
                n266 = And(x=w427, y=w428) -> (x .and. y?=w426:bool)
                n267 = local read "solution"() -> (w425:dbl)
                n268 = Select(t=2.0, s=w426, f=w425) -> (s? t:f=w424:dbl)
                n269 = local write "solution"(w424) -> ()
              }
              frame "X1-2B" {
                n270 = call "turnOffFault3.vi"() -> ()  [unwired: 12 in]
                n271 = local read "solution"() -> (w431:dbl)
                n272 = local read "lab"() -> (w438:dbl)
                n273 = Equal To 0?(x=w431) -> (x = 0?=w436:bool)
                n274 = Equal?(x=w438, y=3.0) -> (x = y?=w437:bool)
                n275 = And(x=w436, y=w437) -> (x .and. y?=w435:bool)
                n276 = local read "solution"() -> (w434:dbl)
                n277 = Select(t=2.0, s=w435, f=w434) -> (s? t:f=w433:dbl)
                n278 = local write "solution"(w433) -> ()
              }
              frame "X1-3B" {
              }
              frame "X1-4B" {
              }
              frame "X1-5B" {
                n279 = call "turnOffFault4.vi"() -> ()  [unwired: 12 in]
                n280 = local read "solution"() -> (w440:dbl)
                n281 = local read "lab"() -> (w447:dbl)
                n282 = Equal To 0?(x=w440) -> (x = 0?=w445:bool)
                n283 = Equal?(x=w447, y=4.0) -> (x = y?=w446:bool)
                n284 = And(x=w445, y=w446) -> (x .and. y?=w444:bool)
                n285 = local read "solution"() -> (w443:dbl)
                n286 = Select(t=2.0, s=w444, f=w443) -> (s? t:f=w442:dbl)
                n287 = local write "solution"(w442) -> ()
              }
              frame "X1-6B" {
              }
              frame "X1-7B" {
              }
              frame "X1-8B" {
              }
              frame "X1-9B" {
              }
              frame "X1-10B" {
              }
              frame "X1-11B" {
              }
              frame "X1-12B" {
              }
              frame "X1-1C" {
              }
              frame "X1-2C" {
              }
              frame "X1-3C" {
              }
              frame "X1-4C" {
              }
              frame "X1-5C" {
              }
              frame "X1-6C" {
              }
              frame "X1-7C" {
              }
              frame "X1-8C" {
              }
              frame "X1-9C" {
              }
              frame "X1-10C" {
                n288 = call "turnOffFault6.vi"() -> ()  [unwired: 12 in]
                n289 = local read "solution"() -> (w449:dbl)
                n290 = local read "lab"() -> (w456:dbl)
                n291 = Equal To 0?(x=w449) -> (x = 0?=w454:bool)
                n292 = Equal?(x=w456, y=6.0) -> (x = y?=w455:bool)
                n293 = And(x=w454, y=w455) -> (x .and. y?=w453:bool)
                n294 = local read "solution"() -> (w452:dbl)
                n295 = Select(t=2.0, s=w453, f=w452) -> (s? t:f=w451:dbl)
                n296 = local write "solution"(w451) -> ()
              }
              frame "X1-11C" {
              }
              frame "X1-12C" {
              }
              frame "X1-1D" {
              }
              frame "X1-2D" {
              }
              frame "X1-3D" {
              }
              frame "X1-4D" {
              }
              frame "X1-5D" {
              }
              frame "X1-6D" {
              }
              frame "X1-7D" {
              }
              frame "X1-8D" {
              }
              frame "X1-9D" {
              }
              frame "X1-10D" {
              }
              frame "X1-11D" {
              }
              frame "X1-12D" {
              }
              frame "PLC-VDC(O/0)" {
              }
              frame "PLC-O/0" {
              }
              frame "PLC-VDC(O/1)" {
                n297 = call "turnOffFault8.vi"() -> ()  [unwired: 12 in]
                n298 = local read "solution"() -> (w458:dbl)
                n299 = local read "lab"() -> (w465:dbl)
                n300 = Equal To 0?(x=w458) -> (x = 0?=w463:bool)
                n301 = Equal?(x=w465, y=8.0) -> (x = y?=w464:bool)
                n302 = And(x=w463, y=w464) -> (x .and. y?=w462:bool)
                n303 = local read "solution"() -> (w461:dbl)
                n304 = Select(t=3.0, s=w462, f=w461) -> (s? t:f=w460:dbl)
                n305 = local write "solution"(w460) -> ()
              }
              frame "PLC-O/1" {
              }
              frame "PLC-VDC(O/2)" {
              }
              frame "PLC-O/2" {
              }
              frame "PLC-VDC(O/3)" {
              }
              frame "PLC-O/3" {
              }
              frame "PLC-DC_COM1" {
                n306 = call "turnOffFault6.vi"() -> ()  [unwired: 12 in]
                n307 = local read "solution"() -> (w467:dbl)
                n308 = local read "lab"() -> (w474:dbl)
                n309 = Equal To 0?(x=w467) -> (x = 0?=w472:bool)
                n310 = Equal?(x=w474, y=6.0) -> (x = y?=w473:bool)
                n311 = And(x=w472, y=w473) -> (x .and. y?=w471:bool)
                n312 = local read "solution"() -> (w470:dbl)
                n313 = Select(t=3.0, s=w471, f=w470) -> (s? t:f=w469:dbl)
                n314 = local write "solution"(w469) -> ()
              }
              frame "PLC-I/0" {
              }
              frame "PLC-I/1" {
              }
              frame "PLC-I/2" {
              }
              frame "PLC-I/3" {
              }
              frame "PLC-DC_COM2" {
              }
              frame "PLC-I/4" {
              }
              frame "PLC-I/5" {
              }
              frame "PLC-I/6" {
              }
              frame "PLC-I/7" {
              }
              frame "Start Button Terminals" {
                n315 = call "turnOffFault1.vi"() -> ()  [unwired: 12 in]
                n316 = local read "solution"() -> (w476:dbl)
                n317 = local read "lab"() -> (w483:dbl)
                n318 = Equal To 0?(x=w476) -> (x = 0?=w481:bool)
                n319 = Equal?(x=w483, y=1.0) -> (x = y?=w482:bool)
                n320 = And(x=w481, y=w482) -> (x .and. y?=w480:bool)
                n321 = local read "solution"() -> (w479:dbl)
                n322 = Select(t=3.0, s=w480, f=w479) -> (s? t:f=w478:dbl)
                n323 = local write "solution"(w478) -> ()
              }
              frame "Stop Button Terminals" {
                n324 = call "turnOffFault3.vi"() -> ()  [unwired: 12 in]
                n325 = local read "solution"() -> (w485:dbl)
                n326 = local read "lab"() -> (w492:dbl)
                n327 = Equal To 0?(x=w485) -> (x = 0?=w490:bool)
                n328 = Equal?(x=w492, y=3.0) -> (x = y?=w491:bool)
                n329 = And(x=w490, y=w491) -> (x .and. y?=w489:bool)
                n330 = local read "solution"() -> (w488:dbl)
                n331 = Select(t=3.0, s=w489, f=w488) -> (s? t:f=w487:dbl)
                n332 = local write "solution"(w487) -> ()
              }
              frame "Auto/Man Terminals" {
              }
              frame "DM1(a0) Terminals" {
              }
              frame "DM2(a1) Terminals" {
                n333 = call "turnOffFault4.vi"() -> ()  [unwired: 12 in]
                n334 = local read "solution"() -> (w494:dbl)
                n335 = local read "lab"() -> (w501:dbl)
                n336 = Equal To 0?(x=w494) -> (x = 0?=w499:bool)
                n337 = Equal?(x=w501, y=4.0) -> (x = y?=w500:bool)
                n338 = And(x=w499, y=w500) -> (x .and. y?=w498:bool)
                n339 = local read "solution"() -> (w497:dbl)
                n340 = Select(t=3.0, s=w498, f=w497) -> (s? t:f=w496:dbl)
                n341 = local write "solution"(w496) -> ()
              }
              frame "DM3(b0) Terminals" {
              }
              frame "DM4(b1) Terminals" {
              }
              frame "DM5(v) Terminals" {
              }
              frame "EL1(A+) Terminals" {
                n342 = call "turnOffFault7.vi"() -> ()  [unwired: 12 in]
                n343 = local read "solution"() -> (w503:dbl)
                n344 = local read "lab"() -> (w510:dbl)
                n345 = Equal To 0?(x=w503) -> (x = 0?=w508:bool)
                n346 = Equal?(x=w510, y=7.0) -> (x = y?=w509:bool)
                n347 = And(x=w508, y=w509) -> (x .and. y?=w507:bool)
                n348 = local read "solution"() -> (w506:dbl)
                n349 = Select(t=3.0, s=w507, f=w506) -> (s? t:f=w505:dbl)
                n350 = local write "solution"(w505) -> ()
              }
              frame "EL2(A-) Terminals" {
              }
              frame "EL3(B+) Terminals" {
              }
              frame "EL4(V+) Terminals" {
              }
            }
          }
        }
      }
      event "Reset Lab": Value Change {
        n351 = event-data() -> ()  [unwired: 1 in, 1 out]
        n352 = case shown="True" "Reset Lab" {
          tunnel: [FALSE ("T button?") w524] -> w512
          frame False {
          }
          frame True {
            n353 = call "resetLabDialog.vi"() -> ("T button?"=w524:bool)  [unwired: 11 in]
            n354 = case shown="True" w524 {
              frame False {
              }
              frame True {
                n355 = flat-sequence {
                  tunnel: [w527] -> w525
                  tunnel: [w529] -> w526
                  tunnel: w525 -> [w529]
                  tunnel: w526 -> [w530]
                  frame #0 {
                    n356 = local read "lab"() -> (w527:dbl)
                    n357 = call "gracefulShutDown.vi"() -> ()  [unwired: 12 in]
                  }
                  frame #1 {
                    n358 = control-ref of="This VI"() -> (w528:refnum<vi>)
                    n359 = invoke class="VI" method="Default Vals.Reinit All"(reference=w528) -> ()  [unwired: 2 in, 3 out]
                  }
                  frame #2 {
                    n360 = local write "lab"(w530) -> ()
                  }
                  frame #3 {
                    n361 = local read "lab"() -> (w532:dbl)
                    n362 = case shown="2" w532 {
                      tunnel: [w533 w534 w535 w536 w537 w538 w539 w540] -> w531
                      frame 1, Default {
                        n363 = call "turnOnFault1.vi"() -> ()  [unwired: 12 in]
                        n364 = call "lab1Text.vi"() -> ("String"=w533:string)  [unwired: 11 in]
                      }
                      frame 2 {
                        n365 = call "turnOnFault2.vi"() -> ()  [unwired: 12 in]
                        n366 = call "lab2Text.vi"() -> ("String"=w534:string)  [unwired: 11 in]
                      }
                      frame 3 {
                        n367 = call "turnOnFault3.vi"() -> ()  [unwired: 12 in]
                        n368 = call "lab3Text.vi"() -> ("String"=w535:string)  [unwired: 11 in]
                      }
                      frame 4 {
                        n369 = call "turnOnFault4.vi"() -> ()  [unwired: 12 in]
                        n370 = call "lab4Text.vi"() -> ("String"=w536:string)  [unwired: 11 in]
                      }
                      frame 5 {
                        n371 = call "turnOnFault5.vi"() -> ()  [unwired: 12 in]
                        n372 = call "lab5Text.vi"() -> ("String"=w537:string)  [unwired: 11 in]
                      }
                      frame 6 {
                        n373 = call "turnOnFault6.vi"() -> ()  [unwired: 12 in]
                        n374 = call "lab6Text.vi"() -> ("String"=w538:string)  [unwired: 11 in]
                      }
                      frame 7 {
                        n375 = call "turnOnFault7.vi"() -> ()  [unwired: 12 in]
                        n376 = call "lab7Text.vi"() -> ("String"=w539:string)  [unwired: 11 in]
                      }
                      frame 8 {
                        n377 = call "turnOnFault8.vi"() -> ()  [unwired: 12 in]
                        n378 = call "lab8Text.vi"() -> ("String"=w540:string)  [unwired: 11 in]
                      }
                    }
                    n379 = local write "Lab:"(w531) -> ()
                  }
                }
              }
            }
          }
        }
        n380 = case shown="True" w512 {
          tunnel: w517 -> [_ w522]
          tunnel: w516 -> [w518 w521]
          tunnel: [w518 w520] -> w515
          frame False {
          }
          frame True {
            n381 = Enqueue Element(queue=w522, element=controls."Reset Lab", error in (no error)=w521) -> (error out=w520:errorcluster)  [unwired: 1 in, 2 out]
          }
        }
      }
      event "Close Lab": Value Change {
        n382 = event-data() -> ()  [unwired: 1 in, 1 out]
        n383 = case shown="True" "Close Lab" {
          tunnel: [FALSE ("true") w549] -> w541
          frame False {
          }
          frame True {
            n384 = local read "Issue Resolved:"() -> (w550:bool)
            n385 = case shown="True" w550 {
              tunnel: [w552 w553] -> w549
              frame False {
                n386 = One Button Dialog(message="You have failed to resolve the issue in this lab.  ") -> (true=w552:bool)  [unwired: 1 in]
              }
              frame True {
                n387 = local read "solution"() -> (w554:dbl)
                n388 = case shown="1, Default" w554 {
                  tunnel: [w555 w557 w559] -> w553
                  frame 1, Default {
                    n389 = One Button Dialog(message="You have succesfully resolved the issue present in this lab.  However, the component that you replaced wasn't broken.  There were alternative solutions to this lab that didn't require the use of your budget.  Please take a screenshot and send it to your instructor.  ") -> (true=w555:bool)  [unwired: 1 in]
                  }
                  frame 2 {
                    n390 = One Button Dialog(message="You have succesfully resolved the issue present in this lab.  However, there was a more accurate alternative solution available.  Please take a screen shot and send it to your instructor.") -> (true=w557:bool)  [unwired: 1 in]
                  }
                  frame 3 {
                    n391 = One Button Dialog(message="You have succesfully resolved the issue present in this lab.  You have found the best possible solution!  Please take a screen shot and send it to your instructor.") -> (true=w559:bool)  [unwired: 1 in]
                  }
                }
              }
            }
          }
        }
        n392 = Enqueue Element(queue=w546, element=controls."Close Lab", error in (no error)=w547) -> (error out=w545:errorcluster)  [unwired: 1 in, 2 out]
      }
    }
    n393 = local read "solution"() -> (w20:dbl)
    n394 = Unbundle By Name(w25) -> ("status"=w23:bool)
    n395 = Not Equal To 0?(x=w20) -> (x != 0?=→"Issue Resolved:":bool)
    n396 = Or(x=w23, y=w22) -> (x .or. y?=w24:bool)
  }
  n397 = while {
    tunnel: w4 -> [w567]
    tunnel: w3 -> [_]
    tunnel: w2 -> [w563]
    shift-right: [w562] -> w1
    shift-left: _ -> [w561]
    stop <- w564 stop-if-true
    n398 = Dequeue Element(queue=w567) -> (element=w566:T5, error out=w565:errorcluster)  [unwired: 2 in, 2 out]
    n399 = Wait (ms)(milliseconds to wait=u32 100 ("millisecond timer value")) -> ()  [unwired: 1 out]
    n400 = case shown="No Error" w565 {
      tunnel: w566 -> [w573 _]
      tunnel: [w572 TRUE] -> w564
      tunnel: w563 -> [w571 _]
      tunnel: [w570 w900] -> w562
      tunnel: w561 -> [w569 w900]
      frame No Error {
        n401 = case shown="\"Initialize\"" w573 {
          tunnel: [FALSE FALSE FALSE FALSE FALSE FALSE FALSE FALSE FALSE FALSE FALSE FALSE FALSE TRUE] -> w572
          tunnel: w571 -> [w575 _ _ _ _ _ _ _ _ _ _ _ _ _]
          tunnel: [w574 w593 w598 w615 w630 w646 w660 w674 w688 w708 w754 w782 w874 w888] -> w570
          tunnel: w569 -> [_ w594 w608 w623 w639 w644 w658 w672 w696 w716 w763 w791 w883 w897]
          frame "Initialize" {
            n402 = case shown="False" w575 {
              tunnel: [w578 w581] -> w574
              frame False {
                n403 = Open/Create/Replace File(file path (use dialog)=path "C:/Users/nolan/Documents/HMI/userLog.txt" ("path"), operation (0:open)=T7."open or create") -> (refnum out=w578:refnum<file>)  [unwired: 4 in, 2 out]
              }
              frame True {
                n404 = Open/Create/Replace File(file path (use dialog)=path "C:/Users/abohman/Desktop/iMEC-HMI/userLog.txt" ("path"), operation (0:open)=T7."open") -> (refnum out=w581:refnum<file>)  [unwired: 4 in, 2 out]
              }
            }
          }
          frame "Start Button" {
            n405 = Set File Position(refnum=w594, from (0:start)=enum16{"start", "end", "current"}."end") -> (refnum out=w592:refnum<file>)  [unwired: 2 in, 1 out]
            n406 = local read "Time Remaining:"() -> (w589:timestamp)
            n407 = local read "Budget:"() -> (w586:dbl)
            n408 = Number To Decimal String(number=w586) -> (decimal integer string=w585:string)  [unwired: 1 in]
            n409 = Format Date/Time String(time format string (%c)="%M:%S", seconds (now)=w589) -> (date/time string=w588:string)  [unwired: 1 in]
            n410 = Concatenate Strings("Start Button," ("string"), w588, ",", w585, "\r") -> (w591:string)
            n411 = Write to Text File(file (use dialog)=w592, text=w591) -> (refnum out=w593:refnum<file>)  [unwired: 2 in, 2 out]
          }
          frame "Stop Button" {
            n412 = Set File Position(refnum=w608, from (0:start)=enum16{"start", "end", "current"}."end") -> (refnum out=w599:refnum<file>)  [unwired: 2 in, 1 out]
            n413 = local read "Time Remaining:"() -> (w605:timestamp)
            n414 = local read "Budget:"() -> (w602:dbl)
            n415 = Number To Decimal String(number=w602) -> (decimal integer string=w601:string)  [unwired: 1 in]
            n416 = Format Date/Time String(time format string (%c)="%M:%S", seconds (now)=w605) -> (date/time string=w604:string)  [unwired: 1 in]
            n417 = Concatenate Strings("Stop Button," ("string"), w604, ",", w601, "\r") -> (w607:string)
            n418 = Write to Text File(file (use dialog)=w599, text=w607) -> (refnum out=w598:refnum<file>)  [unwired: 2 in, 2 out]
          }
          frame "AutoMan Switch" {
            n419 = Set File Position(refnum=w623, from (0:start)=enum16{"start", "end", "current"}."end") -> (refnum out=w614:refnum<file>)  [unwired: 2 in, 1 out]
            n420 = local read "AUTO/MAN"() -> (w612:bool)
            n421 = case shown="False" w612 {
              tunnel: ["Automatic," ("string") "Manual," ("string")] -> w613
              frame False {
              }
              frame True {
              }
            }
            n422 = local read "Time Remaining:"() -> (w621:timestamp)
            n423 = local read "Budget:"() -> (w618:dbl)
            n424 = Number To Decimal String(number=w618) -> (decimal integer string=w617:string)  [unwired: 1 in]
            n425 = Format Date/Time String(time format string (%c)="%M:%S", seconds (now)=w621) -> (date/time string=w620:string)  [unwired: 1 in]
            n426 = Concatenate Strings(w613, w620, ",", w617, "\r") -> (w622:string)
            n427 = Write to Text File(file (use dialog)=w614, text=w622) -> (refnum out=w615:refnum<file>)  [unwired: 2 in, 2 out]
          }
          frame "A Plus Button" {
            n428 = Set File Position(refnum=w639, from (0:start)=enum16{"start", "end", "current"}."end") -> (refnum out=w629:refnum<file>)  [unwired: 2 in, 1 out]
            n429 = local read "Time Remaining:"() -> (w636:timestamp)
            n430 = local read "Budget:"() -> (w633:dbl)
            n431 = Number To Decimal String(number=w633) -> (decimal integer string=w632:string)  [unwired: 1 in]
            n432 = Format Date/Time String(time format string (%c)="%M:%S", seconds (now)=w636) -> (date/time string=w635:string)  [unwired: 1 in]
            n433 = Concatenate Strings("A+ Solenoid," ("string"), w635, ",", w632, "\r") -> (w638:string)
            n434 = Write to Text File(file (use dialog)=w629, text=w638) -> (refnum out=w630:refnum<file>)  [unwired: 2 in, 2 out]
          }
          frame "A Minus Button" {
            n435 = Set File Position(refnum=w644, from (0:start)=enum16{"start", "end", "current"}."end") -> (refnum out=w643:refnum<file>)  [unwired: 2 in, 1 out]
            n436 = local read "Time Remaining:"() -> (w652:timestamp)
            n437 = local read "Budget:"() -> (w649:dbl)
            n438 = Number To Decimal String(number=w649) -> (decimal integer string=w648:string)  [unwired: 1 in]
            n439 = Format Date/Time String(time format string (%c)="%M:%S", seconds (now)=w652) -> (date/time string=w651:string)  [unwired: 1 in]
            n440 = Concatenate Strings("A- Solenoid," ("string"), w651, ",", w648, "\r") -> (w654:string)
            n441 = Write to Text File(file (use dialog)=w643, text=w654) -> (refnum out=w646:refnum<file>)  [unwired: 2 in, 2 out]
          }
          frame "B Plus Button" {
            n442 = Set File Position(refnum=w658, from (0:start)=enum16{"start", "end", "current"}."end") -> (refnum out=w657:refnum<file>)  [unwired: 2 in, 1 out]
            n443 = local read "Time Remaining:"() -> (w666:timestamp)
            n444 = local read "Budget:"() -> (w663:dbl)
            n445 = Number To Decimal String(number=w663) -> (decimal integer string=w662:string)  [unwired: 1 in]
            n446 = Format Date/Time String(time format string (%c)="%M:%S", seconds (now)=w666) -> (date/time string=w665:string)  [unwired: 1 in]
            n447 = Concatenate Strings("B+ Solenoid," ("string"), w665, ",", w662, "\r") -> (w668:string)
            n448 = Write to Text File(file (use dialog)=w657, text=w668) -> (refnum out=w660:refnum<file>)  [unwired: 2 in, 2 out]
          }
          frame "V Plus Button" {
            n449 = Set File Position(refnum=w672, from (0:start)=enum16{"start", "end", "current"}."end") -> (refnum out=w671:refnum<file>)  [unwired: 2 in, 1 out]
            n450 = local read "Time Remaining:"() -> (w680:timestamp)
            n451 = local read "Budget:"() -> (w677:dbl)
            n452 = Number To Decimal String(number=w677) -> (decimal integer string=w676:string)  [unwired: 1 in]
            n453 = Format Date/Time String(time format string (%c)="%M:%S", seconds (now)=w680) -> (date/time string=w679:string)  [unwired: 1 in]
            n454 = Concatenate Strings("V+ Solenoid," ("string"), w679, ",", w676, "\r") -> (w682:string)
            n455 = Write to Text File(file (use dialog)=w671, text=w682) -> (refnum out=w674:refnum<file>)  [unwired: 2 in, 2 out]
          }
          frame "Change View" {
            n456 = Set File Position(refnum=w696, from (0:start)=enum16{"start", "end", "current"}."end") -> (refnum out=w687:refnum<file>)  [unwired: 2 in, 1 out]
            n457 = local read "Tab Control"() -> (w686:T4)
            n458 = case shown="\"Schematic 4\"" w686 {
              tunnel: ["Camera," "Schematic 1," "Schematic 2," "Schematic 3," "Schematic 4,"] -> w685
              frame "Camera", Default {
              }
              frame "Schematic 1" {
              }
              frame "Schematic 2" {
              }
              frame "Schematic 3" {
              }
              frame "Schematic 4" {
              }
            }
            n459 = local read "Time Remaining:"() -> (w694:timestamp)
            n460 = local read "Budget:"() -> (w691:dbl)
            n461 = Number To Decimal String(number=w691) -> (decimal integer string=w690:string)  [unwired: 1 in]
            n462 = Format Date/Time String(time format string (%c)="%M:%S", seconds (now)=w694) -> (date/time string=w693:string)  [unwired: 1 in]
            n463 = Concatenate Strings(w685, w693, ",", w690, "\r") -> (w695:string)
            n464 = Write to Text File(file (use dialog)=w687, text=w695) -> (refnum out=w688:refnum<file>)  [unwired: 2 in, 2 out]
          }
          frame "Acquire Voltage" {
            n465 = Set File Position(refnum=w716, from (0:start)=enum16{"start", "end", "current"}."end") -> (refnum out=w707:refnum<file>)  [unwired: 2 in, 1 out]
            n466 = local read "Segment:"() -> (w705:T3)
            n467 = case shown="\"DC+(Start)\", Default" w705 {
              tunnel: ["DC+(Start) measured," ("string") "PB(Start) measured," ("string") "I/0(Start) measured," ("string") "DC+(Stop) measured," ("string") "PB(Stop) measured," ("string") "I/1(Stop) measured," ("string") "DC+(Auto/Man) measured," ("string") "I/2(Auto/Man) measured," ("string") "DC+(a0) measured," ("string") "I/3(a0) measured," ("string") "DC+(a1) measured," ("string") "I/4(a1) measured," ("string") "DC+(b0) measured," ("string") "I/5(b0) measured," ("string") "DC+(b1) measured," ("string") "I/6(b1) measured," ("string") "DC+(v) measured," ("string") "I/7(v) measured," ("string") "DC+(O/0)(VAC/VDC) measured," ("string") "O/0(EL1A+) measured," ("string") "EL1A+(A1) measured," ("string") "EL1A+(A2) measured," ("string") "DC+(O/1)(VAC/VDC) measured," ("string") "O/1(EL2A-) measured," ("string") "EL2A-(A1) measured," ("string") "EL2A-(A2) measured," ("string") "O/2(EL3B+)(A1) measured," ("string") "EL3B+(A2) measured," ("string") "O/3(EL4V+)(A1) measured," ("string") "EL4V+(A2) measured," ("string") "DC-(DC_COM) measured," ("string") "DC-(0V) measured," ("string")] -> w706
              frame "DC+(Start)", Default {
              }
              frame "PB(Start)" {
              }
              frame "I/0(Start)" {
              }
              frame "DC+(Stop)" {
              }
              frame "PB(Stop)" {
              }
              frame "I/1(Stop)" {
              }
              frame "DC+(Auto/Man)" {
              }
              frame "I/2(Auto/Man)" {
              }
              frame "DC+(a0)" {
              }
              frame "I/3(a0)" {
              }
              frame "DC+(a1)" {
              }
              frame "I/4(a1)" {
              }
              frame "DC+(b0)" {
              }
              frame "I/5(b0)" {
              }
              frame "DC+(b1)" {
              }
              frame "I/6(b1)" {
              }
              frame "DC+(v)" {
              }
              frame "I/7(v)" {
              }
              frame "DC+(O/0)(VAC/VDC)" {
              }
              frame "O/0(EL1A+)" {
              }
              frame "EL1A+(A1)" {
              }
              frame "EL1A+(A2)" {
              }
              frame "DC+(O/1)(VAC/VDC)" {
              }
              frame "O/1(EL2A-)" {
              }
              frame "EL2A-(A1)" {
              }
              frame "EL2A-(A2)" {
              }
              frame "O/2(EL3B+)(A1)" {
              }
              frame "EL3B+(A2)" {
              }
              frame "O/3(EL4V+)(A1)" {
              }
              frame "EL4V+(A2)" {
              }
              frame "DC-(DC_COM)" {
              }
              frame "DC-(0V)" {
              }
            }
            n468 = local read "Time Remaining:"() -> (w714:timestamp)
            n469 = local read "Budget:"() -> (w711:dbl)
            n470 = Number To Decimal String(number=w711) -> (decimal integer string=w710:string)  [unwired: 1 in]
            n471 = Format Date/Time String(time format string (%c)="%M:%S", seconds (now)=w714) -> (date/time string=w713:string)  [unwired: 1 in]
            n472 = Concatenate Strings(w706, w713, ",", w710, "\r") -> (w715:string)
            n473 = Write to Text File(file (use dialog)=w707, text=w715) -> (refnum out=w708:refnum<file>)  [unwired: 2 in, 2 out]
          }
          frame "Replace Component" {
            n474 = Set File Position(refnum=w763, from (0:start)=enum16{"start", "end", "current"}."end") -> (refnum out=w753:refnum<file>)  [unwired: 2 in, 1 out]
            n475 = local read "Component:"() -> (w752:T2)
            n476 = case shown="\"Auto/Man Switch\"" w752 {
              tunnel: ["Start Button Replaced," ("string") "Stop Button Replaced," ("string") "Auto/Man Switch Replaced," ("string") "DM1(a0) Replaced," ("string") "DM2(a1) Replaced," ("string") "DM3(b0) Replaced," ("string") "DM4(b1) Replaced," ("string") "DM5(v) Replaced," ("string") "EL1(A+) Replaced," ("string") "EL2(A-) Replaced," ("string") "EL3(B+) Replaced," ("string") "EL4(V+) Replaced," ("string") "PLC Replaced," ("string")] -> w761
              frame "Start Button", Default {
              }
              frame "Stop Button" {
              }
              frame "Auto/Man Switch" {
              }
              frame "DM1(a0)" {
              }
              frame "DM2(a1)" {
              }
              frame "DM3(b0)" {
              }
              frame "DM4(b1)" {
              }
              frame "DM5(v)" {
              }
              frame "EL1(A+)" {
              }
              frame "EL2(A-)" {
              }
              frame "EL3(B+)" {
              }
              frame "EL4(V+)" {
              }
              frame "PLC" {
              }
            }
            n477 = local read "Time Remaining:"() -> (w760:timestamp)
            n478 = local read "Budget:"() -> (w757:dbl)
            n479 = Number To Decimal String(number=w757) -> (decimal integer string=w756:string)  [unwired: 1 in]
            n480 = Format Date/Time String(time format string (%c)="%M:%S", seconds (now)=w760) -> (date/time string=w759:string)  [unwired: 1 in]
            n481 = Concatenate Strings(w761, w759, ",", w756, "\r") -> (w762:string)
            n482 = Write to Text File(file (use dialog)=w753, text=w762) -> (refnum out=w754:refnum<file>)  [unwired: 2 in, 2 out]
          }
          frame "Tighten Terminal" {
            n483 = Set File Position(refnum=w791, from (0:start)=enum16{"start", "end", "current"}."end") -> (refnum out=w781:refnum<file>)  [unwired: 2 in, 1 out]
            n484 = local read "Terminal:"() -> (w780:T1)
            n485 = case shown="\"X1-1A\", Default" w780 {
              tunnel: ["X1-1A tightened," ("string") "X1-2A tightened," ("string") "X1-3A tightened," ("string") "X1-4A tightened," ("string") "X1-5A tightened," ("string") "X1-6A tightened," ("string") "X1-7A tightened," ("string") "X1-8A tightened," ("string") "X1-9A tightened," ("string") "X1-10A tightened," ("string") "X1-11A tightened," ("string") "X1-12A tightened," ("string") "X1-1B tightened," ("string") "X1-2B tightened," ("string") "X1-3B tightened," ("string") "X1-4B tightened," ("string") "X1-5B tightened," ("string") "X1-6B tightened," ("string") "X1-7B tightened," ("string") "X1-8B tightened," ("string") "X1-9B tightened," ("string") "X1-10B tightened," ("string") "X1-11B tightened," ("string") "X1-12B tightened," ("string") "X1-1C tightened," ("string") "X1-2C tightened," ("string") "X1-3C tightened," ("string") "X1-4C tightened," ("string") "X1-5C tightened," ("string") "X1-6C tightened," ("string") "X1-7C tightened," ("string") "X1-8C tightened," ("string") "X1-9C tightened," ("string") "X1-10C tightened," ("string") "X1-11C tightened," ("string") "X1-12C tightened," ("string") "X1-1D tightened," ("string") "X1-2D tightened," ("string") "X1-3D tightened," ("string") "X1-4D tightened," ("string") "X1-5D tightened," ("string") "X1-6D tightened," ("string") "X1-7D tightened," ("string") "X1-8D tightened," ("string") "X1-9D tightened," ("string") "X1-10D tightened," ("string") "X1-11D tightened," ("string") "X1-12D tightened," ("string") "PLC-VDC(O/0) tightened," ("string") "PLC-O/0 tightened," ("string") "PLC-VDC(O/1) tightened," ("string") "PLC-O/1 tightened," ("string") "PLC-VDC(O/2) tightened," ("string") "PLC-O/2 tightened," ("string") "PLC-VDC(O/3) tightened," ("string") "PLC-O/3 tightened," ("string") "PLC-DC_COM1 tightened," ("string") "PLC-I/0 tightened," ("string") "PLC-I/1 tightened," ("string") "PLC-I/2 tightened," ("string") "PLC-I/3 tightened," ("string") "PLC-DC_COM2 tightened," ("string") "PLC-I/4 tightened," ("string") "PLC-I/5 tightened," ("string") "PLC-I/6 tightened," ("string") "PLC-I/7 tightened," ("string") "Start Button Terminals tightened," ("string") "Stop Button Terminals tightened," ("string") "Auto/Man Terminals tightened," ("string") "DM1(a0) Terminals tightened," ("string") "DM2(a1) Terminals tightened," ("string") "DM3(b0) Terminals tightened," ("string") "DM4(b1) tightened," ("string") "DM5(v) Terminals tightened," ("string") "EL1(A+) Terminals tightened," ("string") "EL2(A-) Terminals tightened," ("string") "EL3(B+) Terminals tightened," ("string") "EL4(V+) Terminals tightened," ("string")] -> w789
              frame "X1-1A", Default {
              }
              frame "X1-2A" {
              }
              frame "X1-3A" {
              }
              frame "X1-4A" {
              }
              frame "X1-5A" {
              }
              frame "X1-6A" {
              }
              frame "X1-7A" {
              }
              frame "X1-8A" {
              }
              frame "X1-9A" {
              }
              frame "X1-10A" {
              }
              frame "X1-11A" {
              }
              frame "X1-12A" {
              }
              frame "X1-1B" {
              }
              frame "X1-2B" {
              }
              frame "X1-3B" {
              }
              frame "X1-4B" {
              }
              frame "X1-5B" {
              }
              frame "X1-6B" {
              }
              frame "X1-7B" {
              }
              frame "X1-8B" {
              }
              frame "X1-9B" {
              }
              frame "X1-10B" {
              }
              frame "X1-11B" {
              }
              frame "X1-12B" {
              }
              frame "X1-1C" {
              }
              frame "X1-2C" {
              }
              frame "X1-3C" {
              }
              frame "X1-4C" {
              }
              frame "X1-5C" {
              }
              frame "X1-6C" {
              }
              frame "X1-7C" {
              }
              frame "X1-8C" {
              }
              frame "X1-9C" {
              }
              frame "X1-10C" {
              }
              frame "X1-11C" {
              }
              frame "X1-12C" {
              }
              frame "X1-1D" {
              }
              frame "X1-2D" {
              }
              frame "X1-3D" {
              }
              frame "X1-4D" {
              }
              frame "X1-5D" {
              }
              frame "X1-6D" {
              }
              frame "X1-7D" {
              }
              frame "X1-8D" {
              }
              frame "X1-9D" {
              }
              frame "X1-10D" {
              }
              frame "X1-11D" {
              }
              frame "X1-12D" {
              }
              frame "PLC-VDC(O/0)" {
              }
              frame "PLC-O/0" {
              }
              frame "PLC-VDC(O/1)" {
              }
              frame "PLC-O/1" {
              }
              frame "PLC-VDC(O/2)" {
              }
              frame "PLC-O/2" {
              }
              frame "PLC-VDC(O/3)" {
              }
              frame "PLC-O/3" {
              }
              frame "PLC-DC_COM1" {
              }
              frame "PLC-I/0" {
              }
              frame "PLC-I/1" {
              }
              frame "PLC-I/2" {
              }
              frame "PLC-I/3" {
              }
              frame "PLC-DC_COM2" {
              }
              frame "PLC-I/4" {
              }
              frame "PLC-I/5" {
              }
              frame "PLC-I/6" {
              }
              frame "PLC-I/7" {
              }
              frame "Start Button Terminals" {
              }
              frame "Stop Button Terminals" {
              }
              frame "Auto/Man Terminals" {
              }
              frame "DM1(a0) Terminals" {
              }
              frame "DM2(a1) Terminals" {
              }
              frame "DM3(b0) Terminals" {
              }
              frame "DM4(b1) Terminals" {
              }
              frame "DM5(v) Terminals" {
              }
              frame "EL1(A+) Terminals" {
              }
              frame "EL2(A-) Terminals" {
              }
              frame "EL3(B+) Terminals" {
              }
              frame "EL4(V+) Terminals" {
              }
            }
            n486 = local read "Time Remaining:"() -> (w788:timestamp)
            n487 = local read "Budget:"() -> (w785:dbl)
            n488 = Number To Decimal String(number=w785) -> (decimal integer string=w784:string)  [unwired: 1 in]
            n489 = Format Date/Time String(time format string (%c)="%M:%S", seconds (now)=w788) -> (date/time string=w787:string)  [unwired: 1 in]
            n490 = Concatenate Strings(w789, w787, ",", w784, "\r") -> (w790:string)
            n491 = Write to Text File(file (use dialog)=w781, text=w790) -> (refnum out=w782:refnum<file>)  [unwired: 2 in, 2 out]
          }
          frame "Reset Lab" {
            n492 = Set File Position(refnum=w883, from (0:start)=enum16{"start", "end", "current"}."end") -> (refnum out=w873:refnum<file>)  [unwired: 2 in, 1 out]
            n493 = local read "Time Remaining:"() -> (w880:timestamp)
            n494 = local read "Budget:"() -> (w877:dbl)
            n495 = Number To Decimal String(number=w877) -> (decimal integer string=w876:string)  [unwired: 1 in]
            n496 = Format Date/Time String(time format string (%c)="%M:%S", seconds (now)=w880) -> (date/time string=w879:string)  [unwired: 1 in]
            n497 = Concatenate Strings("Reset Lab," ("string"), w879, ",", w876, "\r") -> (w882:string)
            n498 = Write to Text File(file (use dialog)=w873, text=w882) -> (refnum out=w874:refnum<file>)  [unwired: 2 in, 2 out]
          }
          frame "Close Lab" {
            n499 = Set File Position(refnum=w897, from (0:start)=enum16{"start", "end", "current"}."end") -> (refnum out=w887:refnum<file>)  [unwired: 2 in, 1 out]
            n500 = local read "Time Remaining:"() -> (w894:timestamp)
            n501 = local read "Budget:"() -> (w891:dbl)
            n502 = Number To Decimal String(number=w891) -> (decimal integer string=w890:string)  [unwired: 1 in]
            n503 = Format Date/Time String(time format string (%c)="%M:%S", seconds (now)=w894) -> (date/time string=w893:string)  [unwired: 1 in]
            n504 = Concatenate Strings("Lab Closed," ("string"), w893, ",", w890, "\r") -> (w896:string)
            n505 = Write to Text File(file (use dialog)=w887, text=w896) -> (refnum out=w888:refnum<file>)  [unwired: 2 in, 2 out]
          }
        }
      }
      frame Error {
      }
    }
  }
  n506 = while {
    tunnel: w3 -> [_]
    stop <- w904 stop-if-true
    n507 = local read "Time Remaining:"() -> (w906:timestamp)
    n508 = Wait (ms)(milliseconds to wait=u32 100) -> ()  [unwired: 1 out]
    n509 = Equal To 0?(x=w906) -> (x = 0?=w905:bool)
    n510 = case shown="False" w905 {
      tunnel: [FALSE w912] -> w903
      frame False {
        n511 = local read "Time Remaining:"() -> (w911:timestamp)
        n512 = Wait (ms)(milliseconds to wait=u32 1000) -> ()  [unwired: 1 out]
        n513 = Decrement(x=w911) -> (x-1=→"Time Remaining:":timestamp)
      }
      frame True {
        w912 = TRUE
        n514 = property on="Close Lab" class="Bool (strict)"("Val(Sgnl)"=w912) -> ()  [unwired: 2 in, 2 out]
      }
    }
    n515 = local read "Close Lab"() -> (w902:bool)
    n516 = Or(x=w903, y=w902) -> (x .or. y?=w904:bool)
  }
  n517 = Close File(refnum=w1) -> ()  [unwired: 1 in, 2 out]
  n518 = Release Queue(queue=w4, error in (no error)=w10) -> ()  [unwired: 1 in, 3 out]
